vi "CRYGraph Intensity Window.vi"() -> ()   [LabVIEW 2013]
uses:
  <vilib>/Utility/miscctls.llb/LVPoint32TypeDef.ctl
  Control/CRYIntensity Property.ctl
  Control/CRYFlag Cluster.ctl
  <vilib>/Utility/miscctls.llb/LVRowAndColumnTypeDef.ctl
  <vilib>/Utility/miscctls.llb/LVPositionTypeDef.ctl
  SubVI/CRYData View Global.vi
  SubVI/CRYMain Sub Window Global.vi
  CRYCurveLibrary/Global/CRYCurve Library Global.vi
panel:
  out "Legend Ref":refnum<vi>
  in  "LoadFinish":bool
  in  "ScaleFitY":bool
  in  "ScaleFitX":bool
  in  "ToolbarUpdate":bool
  in  "OpenProperty":bool
  out "PropertyTab":string
  in  "RampShow":bool
  out "Intensity Property":T1 {"Type" items=["Rectangle"=0, "Hanning"=1, "Hamming"=2, "Blackman-Harris"=3, "Exact Blackman"=4, "Blackman"=5, "Flat Top"=6, "4 Term B-Harris"=7, "7 Term B-Harris"=8, "Low Sidelobe"=9, "Blackman Nuttall"=11, "Triangle"=30, "Bartlett-Hanning"=31, "Bohman"=32, "Parzen"=33, "Welch"=34, "Kaiser"=60, "Dolph-Chebyshev"=61, "Gaussian"=62]}
  in  "PaletteShow":bool
  in  "FitPanes":bool
  out "Graph Ref":refnum<vi>
  out "Repaint Watermark":i32
  out "Event Name":string
  out "ReportDrop":bool
  out "DirectionKey":bool
  out "PreviewGraph Ref":refnum<vi>
  in  "AxisChange":bool
  in  "RemoveOne":bool
  out "ScaleMin":dbl
  out "ScaleMax":dbl
  out "ScrollTick Ref":refnum<vi>
  out "Scrollbar Ref":refnum<vi>
  in  "PreviewShow":bool
  in  "CursorColor":bool
  out "NewCursIdx":u32
  out "Test":string
  in  "OldCursIdx":u32
  out "Queue Name":string
  in  "StateOut":bool
  in  "Cursor Waves":string[](array[string])
  out "Cursor Coords":T2
  in  "CursorPlot":bool
  out "Cursor Ref":refnum<vi>
  in  "CursorShow":bool
  out "IntensityGraph":dbl[][](graph)
  out "Title Name":string
  out "OldRow":i32
  out "TotalPlot":u32
  out "Graph Number":i32
  in  "stop":bool
  out "PreviewGraph":cluster{"xo":dbl, "dx":dbl, dbl[]}[](graph)
  in  "CursorEnabled":bool
  in  "Scrollbar":dbl(c297)
  in  "ScrollTick":dbl(slide) scale=0.0..1.0 scale format="%-#3.2p"
  in  "Cursor":string[][](table)
  in  "LegendShow":bool
  in  "Ramp":u16(ring)
  in  "Legend":i32(listbox)
  in  "GraphType":string
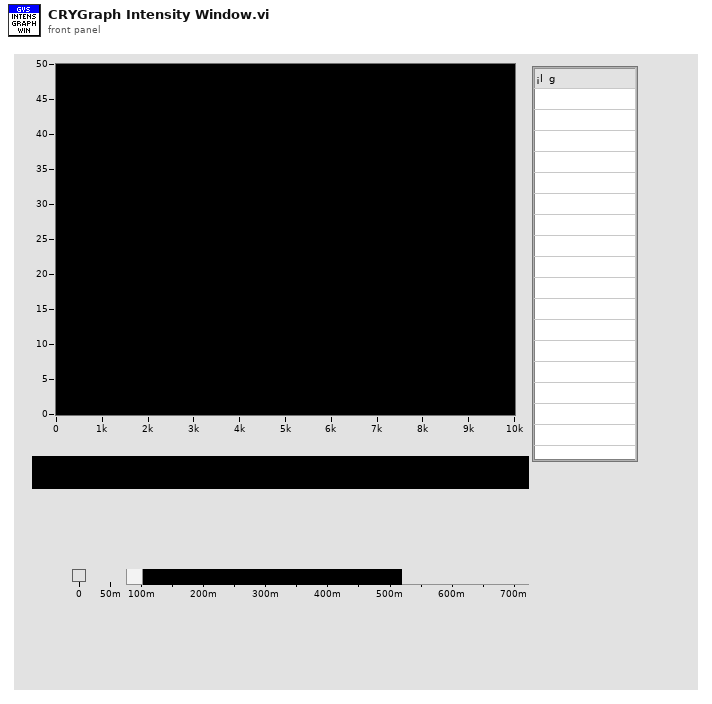
[diagram p1: front panel]
types:
  T1 = typedef "CRYIntensity Property.ctl" = cluster{"Time Steps":i32, "Frequency Bins":i32, "Type":u32, "Length":i32, "Map Type":enum16{"fire", "rainbow", "grey", "inverse grey", "ice", "original"}}
  T2 = typedef "LVPoint32TypeDef.ctl" = cluster{"Horizontal":i32, "Vertical":i32}
  T3 = typedef "CRYFlag Cluster.ctl" = cluster{"LegendShow":bool, "CellClick":bool, "Total Number":bool, "ScaleFitX":bool, "ScaleFitY":bool, "MapModeX":u8, "MapModeY":u8, "CursorShow":bool, "MagnitudeShow":bool, "PreviewShow":bool, "CursorEnabled":bool, "IntensityShow":bool, "PaletteShow":bool, "PhaseShow":bool, "XYShow":bool, "FrequencyShow":bool, "LegendVScrollShow":bool, "FrequencyVScrollShow":bool}
  T4 = typedef "LVPositionTypeDef.ctl" = cluster{"Left":i32, "Top":i32}
  T5 = typedef "LVRowAndColumnTypeDef.ctl" = cluster{"Row":i32, "Column":i32}
  T6 = typedef "CRYGraph Event.ctl" = cluster{"EvenName":string, "TitleName":string, "GraphName":string, "GraphType":string, "Data":variant, "Queue Name":string, "DataView Number":i32}
  T7 = enum16{"fire", "rainbow", "grey", "inverse grey", "ice", "original"}
  T8 = enum16{"No Scaling", "Scale All Objects", "Scale Single Object"}
  T9 = typedef "LVRectTypeDef.ctl" = cluster{"Left":i16, "Top":i16, "Right":i16, "Bottom":i16}
  T10 = typedef "LVBoundsTypeDef.ctl" = cluster{"Width":u32, "Height":u32}
  T11 = typedef "CRYWaveform Cluster.ctl" = cluster{"Waveform":cluster{"X0":dbl, "dX":dbl, "Y":sgl[]}, "X data":u16, "Y data":u16, "Y axis":u16, "X unit":string, "Y unit":string, "Y dB ref":dbl, "display Y":bool, "display X":bool, "Overload?":bool, "Test Info":string, "Step No.":i32, "Name":string, "protected":bool, "Sqc history":string[], "Signal Channel ID":i32, "Plot Settings":cluster{"Color":u32, "Interpolation":u8, "Point Style":u8, "Line Style":u8, "Point Color":u32, "Line Width":u8, "Bar Plot Style":u8, "Fill To":i16}, "AutoProtect":bool}
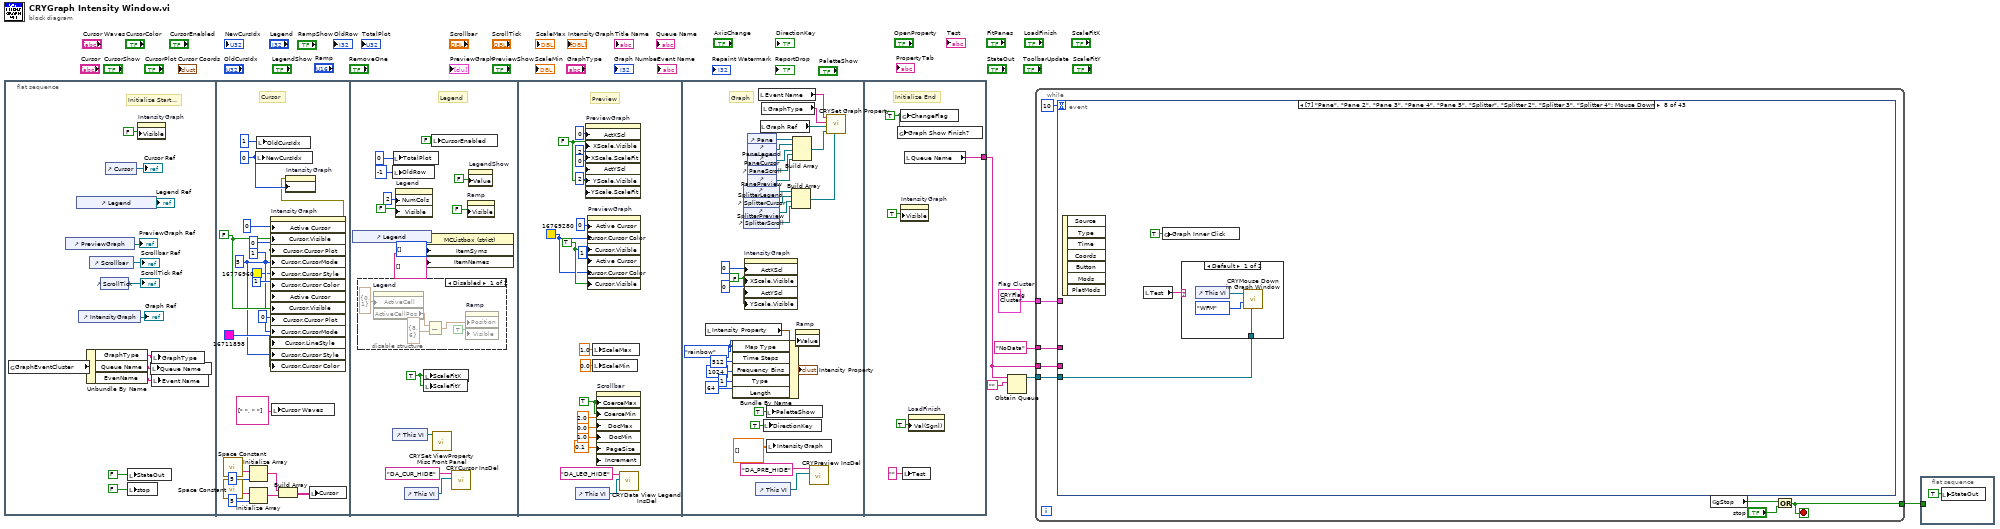
[diagram p0: block diagram]
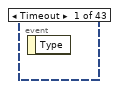
[diagram p3: hidden frame]
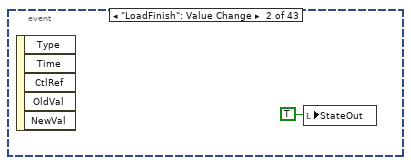
[diagram p4: hidden frame]
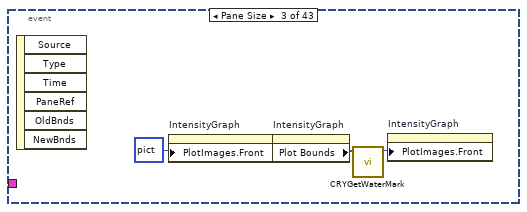
[diagram p5: hidden frame]
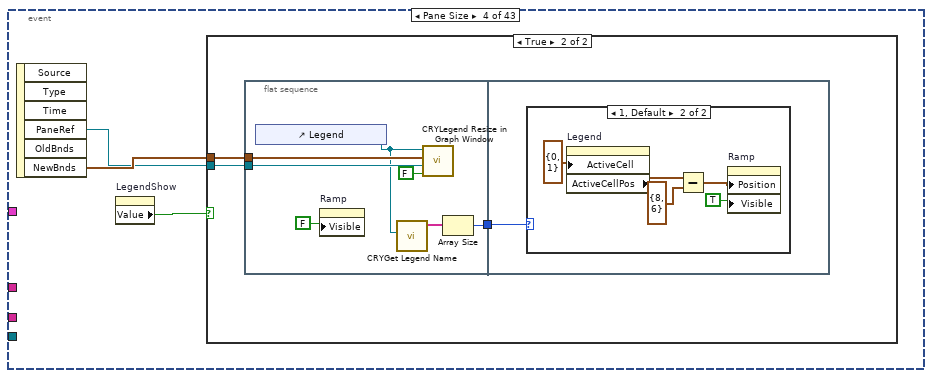
[diagram p6: hidden frame]
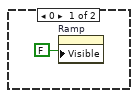
[diagram p8: hidden frame]
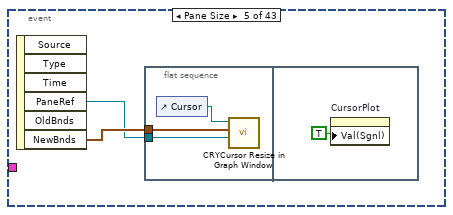
[diagram p9: hidden frame]
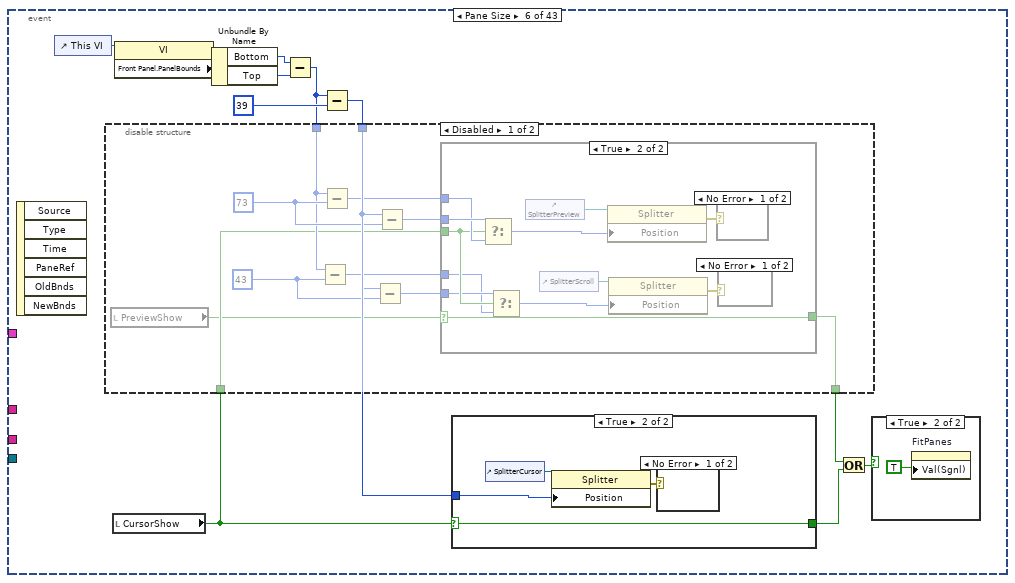
[diagram p10: hidden frame]
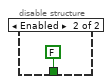
[diagram p14: hidden frame]
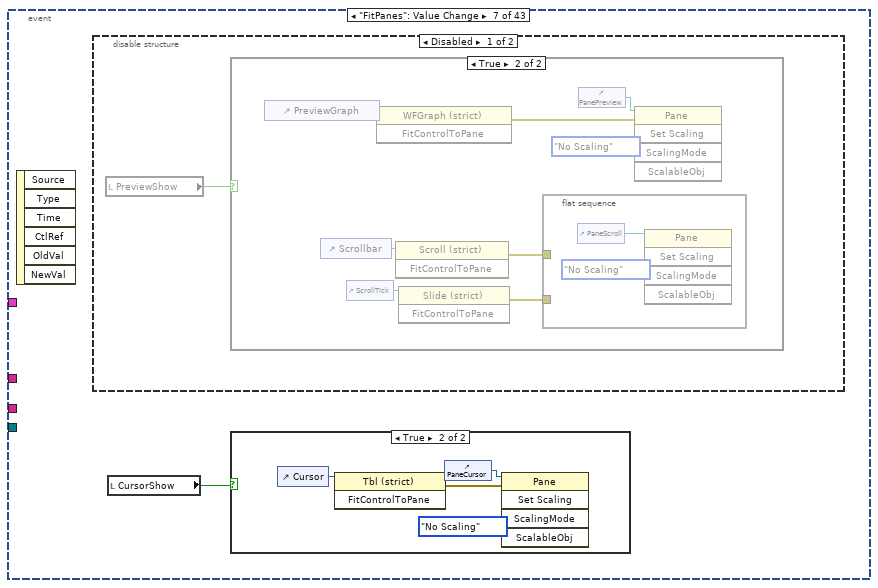
[diagram p18: hidden frame]
diagram:
  w4 = T3 {"LegendShow"=FALSE, "CellClick"=FALSE, "Total Number"=FALSE, "ScaleFitX"=FALSE, "ScaleFitY"=FALSE, "MapModeX"=0, "MapModeY"=0, "CursorShow"=FALSE, "MagnitudeShow"=FALSE, "PreviewShow"=FALSE, "CursorEnabled"=FALSE, "IntensityShow"=FALSE, "PaletteShow"=FALSE, "PhaseShow"=FALSE, "XYShow"=FALSE, "FrequencyShow"=FALSE, "LegendVScrollShow"=FALSE, "FrequencyVScrollShow"=FALSE}  # Flag Cluster
  n1 = flat-sequence {
    tunnel: [w107] -> w2
    frame #0 {
      # "Initialize Start..."
      n2 = global read "CRYData View Global.vi" "GraphEventCluster"() -> (w8:T6)
      n3 = control-ref of="PreviewGraph"() -> (→"PreviewGraph Ref":refnum<vi>)
      n4 = control-ref of="Legend"() -> (→"Legend Ref":refnum<vi>)
      n5 = control-ref of="IntensityGraph"() -> (→"Graph Ref":refnum<vi>)
      n6 = Unbundle By Name(w8) -> ("GraphType"=w10:string, "Queue Name"=w9:string, "EvenName"=w11:string)
      n7 = control-ref of="Scrollbar"() -> (→"Scrollbar Ref":refnum<vi>)
      n8 = control-ref of="ScrollTick"() -> (→"ScrollTick Ref":refnum<vi>)
      n9 = control-ref of="Cursor"() -> (→"Cursor Ref":refnum<vi>)
      n10 = local write "StateOut"(FALSE ("StateOut")) -> ()
      n11 = local write "stop"(FALSE ("stop")) -> ()
      n12 = property on="IntensityGraph" class="IntGraph (strict)"("Visible"=FALSE) -> ()  [unwired: 2 in, 2 out]
      n13 = local write "Queue Name"(w9) -> ()
      n14 = local write "GraphType"(w10) -> ()
      n15 = local write "Event Name"(w11) -> ()
    }
    frame #1 {
      w23 = u32 0 ("Active Cursor")
      w20 = u8 5 ("Cursor.Cursor Style")
      w26 = u32 1 ("Cursor.Cursor Mode")
      w27 = 0 ("Cursor.Cursor Plot")
      w28 = FALSE ("Cursor.Visible")
      # "Cursor"
      n16 = call <vilib>:"Space Constant.vi"() -> ("String"=w32:string)
      n17 = call <vilib>:"Space Constant.vi"() -> ("String"=w37:string)
      n18 = Initialize Array(w32, 5 ("dimension size")) -> (w34:string[])
      n19 = Initialize Array(w37, 5 ("dimension size")) -> (w38:string[])
      n20 = local write "NewCursIdx"(w23) -> ()
      n21 = local write "OldCursIdx"(u32 1 ("OldCursIdx")) -> ()
      n22 = property on="IntensityGraph" class="IntGraph (strict)"("Active Cursor"=u32 0, "Cursor.Visible"=w28, "Cursor.Cursor Plot"=w27, "Cursor.CursorMode"=w26, "Cursor.Cursor Style"=w20, "Cursor.Cursor Color"=u32 16776960, "Active Cursor"=u32 1, "Cursor.Visible"=w28, "Cursor.Cursor Plot"=w27, "Cursor.CursorMode"=w26, "Cursor.LineStyle"=u8 0 ("Cursor.Line Style"), "Cursor.Cursor Style"=w20, "Cursor.Cursor Color"=u32 16711898) -> (error out=w22:errorcluster)  [unwired: 2 in, 1 out]
      n23 = local write "Cursor Waves"(string[] [" ", " "] ("Cursor Waves")) -> ()
      n24 = Build Array(w34, w38) -> (w35:string[][])
      n25 = property on="IntensityGraph" class="IntGraph (strict)"(error in=w22, "Active Cursor"=w23) -> ()  [unwired: 1 in, 2 out]
      n26 = local write "Cursor"(w35) -> ()
    }
    frame #2 {
      w40 = TRUE ("ScaleFitX")
      # "Legend"
      n27 = control-ref of="Legend"() -> (w53:refnum<vi>)
      n28 = disable-structure shown="Disabled" {
        frame Disabled {
          n29 = property on="Legend" class="MCListbox (strict)"("ActiveCell"=T5 {"Row"=0, "Column"=1} ("Active Cell:Active Cell")) -> ("ActiveCellPos"=w54:T4)  [unwired: 2 in, 2 out]
          n30 = Subtract(x=w54, y=T4 {"Left"=8, "Top"=6}) -> (x-y=w57:T4)
          n31 = property on="Ramp" class="Ring (strict)"("Position"=w57, "Visible"=TRUE) -> ()  [unwired: 2 in, 2 out]
        }
        frame Enabled {
        }
      }
      n32 = local write "OldRow"(-1 ("OldRow 2")) -> ()
      n33 = control-ref of="This VI"() -> (w42:refnum<vi>)
      n34 = local write "TotalPlot"(u32 0 ("TotalPlot")) -> ()
      n35 = property on="Legend" class="MCListbox (strict)"("NumCols"=u32 2 ("Number of Columns"), "Visible"=FALSE) -> ()  [unwired: 2 in, 2 out]
      n36 = control-ref of="This VI"() -> (w44:refnum<vi>)
      n37 = local write "ScaleFitX"(w40) -> ()
      n38 = local write "ScaleFitY"(w40) -> ()
      n39 = property on="Property Node" class="MCListbox (strict)"(reference=w53, "ItemSyms"=i32[] [] ("Item Symbols"), "ItemNames"=string[][] [] ("Item Names")) -> ()  [unwired: 1 in, 2 out]
      n40 = local write "CursorEnabled"(FALSE ("CursorEnabled")) -> ()
      n41 = call "CRYSet ViewProperty Misc Front Panel.vi"("Vi Ref"=w42) -> ()  [unwired: 11 in]
      n42 = call "CRYCursor InsDel.vi"("Graph VI Ref"=w44, "sAction"="DA_CUR_HIDE" ("Action Type")) -> ()  [unwired: 10 in]
      n43 = property on="Ramp" class="Ring (strict)"("Visible"=FALSE) -> ()  [unwired: 2 in, 2 out]
      n44 = property on="LegendShow" class="Bool (strict)"("Value"=FALSE ("Visible")) -> ()  [unwired: 2 in, 2 out]
    }
    frame #3 {
      w64 = u32 16769280
      w65 = TRUE ("Cursor.Visible")
      w60 = FALSE ("X Scale.Visible")
      w76 = TRUE ("Coerce Maximum Value")
      # "Preview"
      n45 = control-ref of="This VI"() -> (w62:refnum<vi>)
      n46 = property on="PreviewGraph" class="WFGraph (strict)"("ActXScl"=0 ("Active X Scale"), "XScale.Visible"=w60, "XScale.ScaleFit"=u8 2 ("X Scale.Scale Fit"), "ActYScl"=0 ("Active Y Scale"), "YScale.Visible"=w60, "YScale.ScaleFit"=u8 2 ("Y Scale.Scale Fit")) -> ()  [unwired: 2 in, 2 out]
      n47 = property on="PreviewGraph" class="WFGraph (strict)"("Active Cursor"=u32 0, "Cursor.Cursor Color"=w64, "Cursor.Visible"=w65, "Active Cursor"=u32 1, "Cursor.Cursor Color"=w64, "Cursor.Visible"=w65) -> ()  [unwired: 2 in, 2 out]
      n48 = local write "ScaleMax"(1.0 ("ScaleMax")) -> ()
      n49 = local write "ScaleMin"(0.0 ("ScaleMin")) -> ()
      n50 = property on="Scrollbar" class="Scroll (strict)"("CoerceMax"=w76, "CoerceMin"=w76, "DocMax"=2.0 ("Doc Max"), "DocMin"=0.0 ("Doc Min"), "PageSize"=1.0 ("Page Size"), "Increment"=0.1) -> ()  [unwired: 2 in, 2 out]
      n51 = call "CRYData View Legend InsDel.vi"("Graph VI Ref"=w62, "sAction"="DA_LEG_HIDE" ("Action Type")) -> ()  [unwired: 2 in, 8 out]
    }
    frame #4 {
      w77 = FALSE ("X Scale.Visible")
      w81 = T7."rainbow" ("Map Type")
      # "Graph"
      n52 = local read "Intensity Property"() -> (w87:T1)
      n53 = Bundle By Name(cluster=w87, "Map Type"=w81, "Time Steps"=512, "Frequency Bins"=1024, "Type"=u32 1, "Length"=64) -> (→"Intensity Property":T1)
      n54 = control-ref of="SplitterLegend"() -> (w103:refnum<vi>)
      n55 = control-ref of="SplitterCursor"() -> (w102:refnum<vi>)
      n56 = control-ref of="SplitterPreview"() -> (w101:refnum<vi>)
      n57 = control-ref of="SplitterScroll"() -> (w100:refnum<vi>)
      n58 = property on="IntensityGraph" class="IntGraph (strict)"("ActXScl"=0 ("Active X Scale"), "XScale.Visible"=w77, "ActYScl"=0 ("Active Y Scale"), "YScale.Visible"=w77) -> ()  [unwired: 2 in, 2 out]
      n59 = control-ref of="Pane"() -> (w99:refnum<vi>)
      n60 = control-ref of="PaneLegend"() -> (w95:refnum<vi>)
      n61 = control-ref of="PaneCursor"() -> (w98:refnum<vi>)
      n62 = control-ref of="PaneScroll"() -> (w97:refnum<vi>)
      n63 = control-ref of="PanePreview"() -> (w96:refnum<vi>)
      n64 = control-ref of="This VI"() -> (w104:refnum<vi>)
      n65 = local read "Event Name"() -> (w89:string)
      n66 = local read "Graph Ref"() -> (w91:refnum<vi>)
      n67 = local read "GraphType"() -> (w90:string)
      n68 = local write "DirectionKey"(TRUE ("ScanCode")) -> ()
      n69 = local write "PaletteShow"(TRUE ("PaletteShow")) -> ()
      n70 = local write "IntensityGraph"(dbl[][] [] ("Graph")) -> ()
      n71 = Build Array(w103, w102, w101, w100) -> (w93:refnum<vi>[])
      n72 = Build Array(w99, w95, w98, w97, w96) -> (w94:refnum<vi>[])
      n73 = property on="Ramp" class="Ring (strict)"("Value"=w81) -> ()  [unwired: 2 in, 2 out]
      n74 = call "CRYPreview InsDel.vi"("Graph VI Ref"=w104, "sAction"="DA_PRE_HIDE" ("Action Type")) -> ()  [unwired: 10 in]
      n75 = call "CRYSet Graph Property.vi"("Splitters"=w93, "Panes"=w94, "Graph Ref"=w91, "Graph Type"=w90, "Event Name"=w89) -> ()  [unwired: 7 in]
    }
    frame #5 {
      w110 = TRUE ("ChangeFlag")
      # "Initialize End"
      n76 = global write "CRYData View Global.vi" "Graph Show Finish?"(w110) -> ()
      n77 = global write "CRYData View Global.vi" "ChangeFlag"(w110) -> ()
      n78 = property on="IntensityGraph" class="IntGraph (strict)"("Visible"=TRUE) -> ()  [unwired: 2 in, 2 out]
      n79 = local write "Test"("" ("Test")) -> ()
      n80 = local read "Queue Name"() -> (w107:string)
      n81 = property on="LoadFinish" class="Bool (strict)"("Val(Sgnl)"=TRUE ("Value (Signaling)")) -> ()  [unwired: 2 in, 2 out]
    }
  }
  n82 = Obtain Queue(name (unnamed)=w2, element data type="") -> (queue out=w6:refnum<queue>)  [unwired: 3 in, 2 out]
  n83 = while {
    tunnel: w6 -> [w118]
    tunnel: w4 -> [w116]
    tunnel: "NoData" ("input 2") -> [w113]
    tunnel: w2 -> [w112]
    tunnel: [w111] -> w1
    stop <- w111 stop-if-true
    n84 = event shown="[7] \"Pane\", \"Pane 2\", \"Pane 3\", \"Pane 4\", \"Pane 5\", \"Splitter\", \"Splitter 2\", \"Splitter 3\", \"Splitter 4\": Mouse Down" {
      selector: _ -> [_ _ _ _ _ _ _ _ _ _ _ _ _ _ _ _ _ _ _ _ _ _ _ _ _ _ _ _ _ _ _ _ _ _ _ _ _ _ _ _ _ _ _]
      dyn-events: _ -> [_ _ _ _ _ _ _ _ _ _ _ _ _ _ _ _ _ _ _ _ _ _ _ _ _ _ _ _ _ _ _ _ _ _ _ _ _ _ _ _ _ _ _]
      timeout: 10 -> [_ _ _ _ _ _ _ _ _ _ _ _ _ _ _ _ _ _ _ _ _ _ _ _ _ _ _ _ _ _ _ _ _ _ _ _ _ _ _ _ _ _ _]
      tunnel: w118 -> [_ _ _ _ _ _ _ w210 _ w243 _ w373 _ w410 _ _ _ _ _ _ _ _ _ _ w556 _ _ _ _ _ _ w643 _ _ w656 _ _ _ _ _ _ _ _]
      tunnel: w116 -> [_ _ _ _ _ _ _ _ w227 _ w355 _ w395 _ _ _ _ _ _ _ _ _ _ _ _ _ _ _ _ _ _ _ _ _ _ _ _ _ _ _ _ _ _]
      tunnel: w113 -> [_ _ _ _ _ _ _ _ _ w245 _ _ _ w409 _ _ _ _ _ _ _ _ _ _ _ _ _ _ _ _ _ _ _ _ _ _ _ _ _ _ _ _ _]
      tunnel: w112 -> [_ _ _ _ _ _ _ _ w220 w244 _ _ _ _ _ _ _ _ _ _ _ _ _ _ _ _ _ _ _ _ _ _ _ _ _ _ _ _ _ _ _ _ _]
      event Timeout {
        n85 = event-data() -> ()  [unwired: 2 out]
      }
      event "LoadFinish": Value Change {
        n86 = event-data() -> ()  [unwired: 6 out]
        n87 = local write "StateOut"(TRUE ("StateOut")) -> ()
      }
      event Pane Size {
        n88 = event-data() -> ()  [unwired: 7 out]
        n89 = property on="IntensityGraph" class="IntGraph (strict)"("PlotImages.Front"=picture data[5B] ("Plot Images:Front")) -> (error out=w120:errorcluster)  [unwired: 2 in, 1 out]
        n90 = property on="IntensityGraph" class="IntGraph (strict)"(error in=w120) -> ("Plot Bounds"=w122:T9)  [unwired: 1 in, 2 out]
        n91 = call "CRYGetWaterMark.vi"("Plot Area Bounds"=w122) -> ("WaterMark Image"=w121:picture)  [unwired: 3 in, 7 out]
        n92 = property on="IntensityGraph" class="IntGraph (strict)"("PlotImages.Front"=w121) -> ()  [unwired: 2 in, 2 out]
      }
      event Pane Size {
        n93 = event-data() -> ("PaneRef"=w125:refnum<vi>, "NewBnds"=w126:T9)  [unwired: 5 out]
        n94 = property on="LegendShow" class="Bool (strict)"() -> ("Value"=w124:bool)  [unwired: 2 in, 2 out]
        n95 = case shown="True" w124 {
          tunnel: w126 -> [_ w128]
          tunnel: w125 -> [_ w127]
          frame False {
          }
          frame True {
            n96 = flat-sequence {
              tunnel: w128 -> [w136]
              tunnel: w127 -> [w135]
              tunnel: [w131] -> w129
              tunnel: w129 -> [w137]
              frame #0 {
                n97 = control-ref of="Legend"() -> (w132:refnum<vi>)
                n98 = property on="Ramp" class="Ring (strict)"("Visible"=FALSE) -> ()  [unwired: 2 in, 2 out]
                n99 = call "CRYGet Legend Name.vi"("MCListbox Refnum"=w132) -> ("Names Out"=w133:string[])  [unwired: 10 in]
                n100 = call "CRYLegend Resize in Graph Window.vi"("VScrollShow"=FALSE, "Pane Ref"=w135, "input cluster"=w136, "Legend"=w132) -> ()  [unwired: 8 out]
                n101 = Array Size(array=w133) -> (size(s)=w131:i32)
              }
              frame #1 {
                n102 = case shown="1, Default" w137 {
                  frame 0 {
                    n103 = property on="Ramp" class="Ring (strict)"("Visible"=FALSE) -> ()  [unwired: 2 in, 2 out]
                  }
                  frame 1, Default {
                    n104 = property on="Legend" class="MCListbox (strict)"("ActiveCell"=T5 {"Row"=0, "Column"=1} ("Active Cell:Active Cell")) -> ("ActiveCellPos"=w143:T4)  [unwired: 2 in, 2 out]
                    n105 = Subtract(x=w143, y=T4 {"Left"=8, "Top"=6}) -> (x-y=w141:T4)
                    n106 = property on="Ramp" class="Ring (strict)"("Position"=w141, "Visible"=TRUE) -> ()  [unwired: 2 in, 2 out]
                  }
                }
              }
            }
          }
        }
      }
      event Pane Size {
        n107 = event-data() -> ("PaneRef"=w144:refnum<vi>, "NewBnds"=w145:T9)  [unwired: 5 out]
        n108 = flat-sequence {
          tunnel: w145 -> [w148]
          tunnel: w144 -> [w146]
          frame #0 {
            n109 = control-ref of="Cursor"() -> (w147:refnum<vi>)
            n110 = call "CRYCursor Resize in Graph Window.vi"("Pane Ref"=w146, "input cluster"=w148, "Graph Cursor Ref"=w147) -> ()  [unwired: 9 in]
          }
          frame #1 {
            n111 = property on="CursorPlot" class="Bool (strict)"("Val(Sgnl)"=TRUE ("Value (Signaling)")) -> ()  [unwired: 2 in, 2 out]
          }
        }
      }
      event Pane Size {
        n112 = event-data() -> ()  [unwired: 7 out]
        n113 = control-ref of="This VI"() -> (w153:refnum<vi>)
        n114 = local read "CursorShow"() -> (w150:bool)
        n115 = property class="VI"(reference=w153) -> ("Front Panel.PanelBounds"=w154:T9)  [unwired: 1 in, 2 out]
        n116 = Unbundle By Name(w154) -> ("Bottom"=w151:i16, "Top"=w152:i16)
        n117 = Subtract(x=w151, y=w152) -> (x-y=w155:i16)
        n118 = Subtract(x=w155, y=39) -> (x-y=w160:i32)
        n119 = disable-structure shown="Disabled" {
          disable-tunnel: w160 -> [w168 _]
          disable-tunnel: [w166 FALSE] -> w156
          disable-tunnel: w155 -> [w163 _]
          disable-tunnel: w150 -> [w162 _]
          frame Disabled {
            w169 = 43
            w167 = 73
            n120 = local read "PreviewShow"() -> (w161:bool)
            n121 = Subtract(x=w163, y=w169) -> (x-y=w165:i32)
            n122 = Subtract(x=w163, y=w167) -> (x-y=w164:i32)
            n123 = Subtract(x=w168, y=w169) -> (x-y=w171:i32)
            n124 = Subtract(x=w168, y=w167) -> (x-y=w170:i32)
            n125 = case shown="True" w161 {
              selector: w161 -> [w172 w182]
              tunnel: w164 -> [_ w180]
              tunnel: w165 -> [_ w176]
              tunnel: [w172 w182] -> w166
              tunnel: w162 -> [_ w178]
              tunnel: w170 -> [_ w181]
              tunnel: w171 -> [_ w177]
              frame False {
              }
              frame True {
                n126 = Select(t=w181, s=w178, f=w180) -> (s? t:f=w179:i32)
                n127 = Select(t=w177, s=w178, f=w176) -> (s? t:f=w175:i32)
                n128 = control-ref of="SplitterPreview"() -> (w174:refnum<vi>)
                n129 = control-ref of="SplitterScroll"() -> (w173:refnum<vi>)
                n130 = property class="Splitter"(reference=w174, "Position"=w179) -> (error out=w184:errorcluster)  [unwired: 1 in, 1 out]
                n131 = property class="Splitter"(reference=w173, "Position"=w175) -> (error out=w183:errorcluster)  [unwired: 1 in, 1 out]
                n132 = case shown="No Error" w184 {
                  frame No Error {
                  }
                  frame Error {
                  }
                }
                n133 = case shown="No Error" w183 {
                  frame No Error {
                  }
                  frame Error {
                  }
                }
              }
            }
          }
          frame Enabled {
          }
        }
        n134 = case shown="True" w150 {
          selector: w150 -> [w187 w189]
          tunnel: w160 -> [_ w191]
          tunnel: [w187 w189] -> w157
          frame False {
          }
          frame True {
            n135 = control-ref of="SplitterCursor"() -> (w188:refnum<vi>)
            n136 = property class="Splitter"(reference=w188, "Position"=w191) -> (error out=w190:errorcluster)  [unwired: 1 in, 1 out]
            n137 = case shown="No Error" w190 {
              frame No Error {
              }
              frame Error {
              }
            }
          }
        }
        n138 = Or(x=w156, y=w157) -> (x .or. y?=w158:bool)
        n139 = case shown="True" w158 {
          frame False {
          }
          frame True {
            n140 = property on="FitPanes" class="Bool (strict)"("Val(Sgnl)"=TRUE ("Value (Signaling)")) -> ()  [unwired: 2 in, 2 out]
          }
        }
      }
      event "FitPanes": Value Change {
        n141 = event-data() -> ()  [unwired: 7 out]
        n142 = disable-structure shown="Disabled" {
          frame Disabled {
            n143 = local read "PreviewShow"() -> (w193:bool)
            n144 = case shown="True" w193 {
              frame False {
              }
              frame True {
                n145 = control-ref of="PreviewGraph"() -> (w200:refnum<vi>)
                n146 = control-ref of="Scrollbar"() -> (w199:refnum<vi>)
                n147 = control-ref of="ScrollTick"() -> (w198:refnum<vi>)
                n148 = invoke class="WFGraph (strict)" method="FitControlToPane"(reference=w200) -> (error out=w197:errorcluster)  [unwired: 2 in, 2 out]
                n149 = invoke class="Scroll (strict)" method="FitControlToPane"(reference=w199) -> (error out=w196:errorcluster)  [unwired: 2 in, 2 out]
                n150 = invoke class="Slide (strict)" method="FitControlToPane"(reference=w198) -> (error out=w195:errorcluster)  [unwired: 2 in, 2 out]
                n151 = flat-sequence {
                  tunnel: w196 -> [_]
                  tunnel: w195 -> [_]
                  frame #0 {
                    n152 = control-ref of="PaneScroll"() -> (w202:refnum<vi>)
                    n153 = invoke class="Pane" method="Set Scaling"(reference=w202, "ScalingMode"=T8."No Scaling" ("Scaling Mode")) -> ()  [unwired: 3 in, 5 out]
                  }
                }
                n154 = control-ref of="PanePreview"() -> (w194:refnum<vi>)
                n155 = invoke class="Pane" method="Set Scaling"(reference=w194, error in=w197, "ScalingMode"=T8."No Scaling" ("Scaling Mode")) -> ()  [unwired: 2 in, 5 out]
              }
            }
          }
          frame Enabled {
          }
        }
        n156 = local read "CursorShow"() -> (w192:bool)
        n157 = case shown="True" w192 {
          frame False {
          }
          frame True {
            n158 = control-ref of="Cursor"() -> (w207:refnum<vi>)
            n159 = invoke class="Tbl (strict)" method="FitControlToPane"(reference=w207) -> (error out=w206:errorcluster)  [unwired: 2 in, 2 out]
            n160 = control-ref of="PaneCursor"() -> (w204:refnum<vi>)
            n161 = invoke class="Pane" method="Set Scaling"(reference=w204, error in=w206, "ScalingMode"=T8."No Scaling" ("Scaling Mode")) -> ()  [unwired: 2 in, 5 out]
          }
        }
      }
      event Mouse Down {
        n162 = event-data() -> ()  [unwired: 8 out]
        n163 = local read "Test"() -> (w209:string)
        n164 = global write "CRYCurve Library Global.vi" "Graph Inner Click"(TRUE ("Graph Inner Click")) -> ()
        n165 = case shown="Default" w209 {
          tunnel: w210 -> [w213 _]
          frame Default {
            n166 = control-ref of="This VI"() -> (w211:refnum<vi>)
            n167 = call "CRYMouse Down in Graph Window.vi"("Queue"=w213, "Selected Type"=enum16{"Curves", "Values", "Results", "WFM"}."WFM" ("Type"), "pGraph VI In"=w211) -> ()  [unwired: 3 in, 6 out]
          }
          frame "Test" {
          }
        }
      }
      event Shortcut Menu Activation? {
        n168 = event-data() -> ("MenuRef"=w229:refnum<k9>)  [unwired: 7 out]
        n169 = property on="IntensityGraph" class="IntGraph (strict)"() -> ("XScale.Mapping Mode"=w225:u8, "YScale.Mapping Mode"=w224:u8)  [unwired: 2 in, 2 out]
        n170 = local read "CursorEnabled"() -> (w222:bool)
        n171 = local read "LegendShow"() -> (w228:bool)
        n172 = local read "PreviewShow"() -> (w221:bool)
        n173 = local read "CursorShow"() -> (w223:bool)
        n174 = local read "PaletteShow"() -> (w216:bool)
        n175 = local read "ScaleFitX"() -> (w215:bool)
        n176 = local read "ScaleFitY"() -> (w214:bool)
        n177 = Bundle By Name(cluster=w227, "LegendShow"=w228, "ScaleFitX"=w215, "ScaleFitY"=w214, "MapModeX"=w225, "MapModeY"=w224, "CursorShow"=w223, "PreviewShow"=w221, "CursorEnabled"=w222, "PaletteShow"=w216) -> (w226:T3)
        n178 = local read "Test"() -> (w217:string)
        n179 = case shown="Default" w217 {
          tunnel: w220 -> [_ w235]
          tunnel: ["" ("sData Out") w234] -> w219
          tunnel: [TRUE ("bResult Out") w233] -> w218
          frame "Test" {
          }
          frame Default {
            n180 = local read "Graph Number"() -> (w232:i32)
            n181 = call "CRYGraph View Socket Client.vi"("sOption"="MENUOPTION", "nData"=w232, "sData"=w235, "sAction"="GET_GRAPHDATA") -> ("bResult Out"=w233:bool, "sData Out"=w234:string)  [unwired: 4 in, 2 out]
          }
        }
        n182 = case shown="True" w218 {
          tunnel: w229 -> [_ w242]
          tunnel: w226 -> [_ w240]
          tunnel: w219 -> [_ w239]
          frame False {
          }
          frame True {
            n183 = control-ref of="This VI"() -> (w238:refnum<vi>)
            n184 = call "CRYGraph Window Menu.vi"("MenuOption"=w239, "pGraph VI"=w238, "Flag Cluster"=w240, "Type"="INTENSITY", "Runtime Menu Ref In"=w242) -> ()  [unwired: 7 out]
          }
        }
        n185 = event-data() -> ()  [unwired: 1 in, 2 out]
      }
      event Shortcut Menu Selection (User) {
        n186 = event-data() -> ("ItemTag"=w246:string)  [unwired: 8 out]
        n187 = case shown="\"DA_SCALE_X_A\", \"DA_SCALE_X_L\", \"DA_SCALE_Y_A\", \"DA_SCALE_Y_L\"" w246 {
          selector: w246 -> [w248 _ w325 w351 _]
          tunnel: w245 -> [_ _ w319 _ _]
          tunnel: w244 -> [_ _ _ _ _]
          tunnel: w243 -> [_ _ w317 _ _]
          frame "DA_SCALE_X_A", "DA_SCALE_X_L", "DA_SCALE_Y_A", "DA_SCALE_Y_L" {
            n188 = case shown="\"DA_SCALE_X_A\", Default" w248 {
              selector: w248 -> [w252 w298 w299 w309]
              tunnel: [w252 w298 w299 w309] -> w247
              frame "DA_SCALE_X_A", Default {
                n189 = local read "ScaleFitX"() -> (w251:bool)
                n190 = Not(x=w251) -> (.not. x?=w250:bool)
                n191 = local write "ScaleFitX"(w250) -> ()
                n192 = Select(t=u8 2, s=w250, f=u8 0) -> (s? t:f=w253:u8)
                n193 = property on="IntensityGraph" class="IntGraph (strict)"("XScale.ScaleFit"=w253) -> (error out=w254:errorcluster)  [unwired: 2 in, 1 out]
                n194 = disable-structure shown="Disabled" {
                  disable-tunnel: w254 -> [w258 _]
                  disable-tunnel: w253 -> [w257 _]
                  frame Disabled {
                    n195 = property on="PreviewGraph" class="WFGraph (strict)"("XScale.ScaleFit"=w257) -> ()  [unwired: 2 in, 2 out]
                    n196 = case shown="2" w257 {
                      tunnel: w258 -> [_ _]
                      frame Default {
                      }
                      frame 2 {
                        n197 = property on="IntensityGraph" class="IntGraph (strict)"() -> ("XScale.Maximum"=w287:dbl, "XScale.Minimum"=w288:dbl)  [unwired: 2 in, 2 out]
                        n198 = property on="PreviewGraph" class="WFGraph (strict)"() -> ("XScale.Maximum"=w268:dbl, "XScale.Minimum"=w262:dbl)  [unwired: 2 in, 2 out]
                        n199 = Greater?(x=w262, y=w288) -> (0:w289:bool)
                        n200 = Less?(x=w268, y=w287) -> (x < y?=w286:bool)
                        n201 = Subtract(x=w268, y=w262) -> (x-y=w267:dbl)
                        n202 = Select(t=w268, s=w286, f=w287) -> (s? t:f=w263:dbl)
                        n203 = Select(t=w262, s=w289, f=w288) -> (s? t:f=w264:dbl)
                        n204 = Subtract(x=w264, y=w262) -> (x-y=w261:dbl)
                        n205 = Subtract(x=w263, y=w262) -> (x-y=w260:dbl)
                        n206 = property on="PreviewGraph" class="WFGraph (strict)"("Active Cursor"=u32 0, "Cursor.Cursor X"=w264, "Active Cursor"=u32 1, "Cursor.Cursor X"=w263) -> (error out=w285:errorcluster)  [unwired: 2 in, 1 out]
                        n207 = Divide(x=w261, y=w267) -> (x/y=w265:dbl)
                        n208 = Divide(x=w260, y=w267) -> (x/y=w266:dbl)
                        n209 = property on="Scrollbar" class="Scroll (strict)"() -> ("DocMax"=w274:dbl, "PageSize"=w280:dbl)  [unwired: 2 in, 2 out]
                        n210 = Subtract(x=w265, y=w266) -> (x-y=w272:dbl)
                        n211 = flat-sequence {
                          tunnel: w285 -> [_]
                          frame #0 {
                            n212 = control-ref of="This VI"() -> (w291:refnum<vi>)
                            n213 = call "CRYPlot Wave Graph Preview.vi"("sOption"="Move", "Graph VI Ref"=w291) -> ()  [unwired: 10 in]
                          }
                        }
                        n214 = Divide(x=w280, y=w272) -> (x/y=w271:dbl)
                        n215 = local read "ScaleMax"() -> (w270:dbl)
                        n216 = local read "ScaleMin"() -> (w269:dbl)
                        n217 = Add(x=w274, y=w271) -> (x+y=w273:dbl)
                        n218 = property on="Scrollbar" class="Scroll (strict)"("DocMin"=w273) -> ("DocMax"=w282:dbl, "DocMin"=w281:dbl)  [unwired: 2 in, 2 out]
                        n219 = Subtract(x=w270, y=w269) -> (x-y=w259:dbl)
                        n220 = Subtract(x=w265, y=w269) -> (x-y=w275:dbl)
                        n221 = Subtract(x=w282, y=w281) -> (x-y=w276:dbl)
                        n222 = Multiply(x=w275, y=w276) -> (x*y=w277:dbl)
                        n223 = Divide(x=w277, y=w259) -> (x/y=w278:dbl)
                        n224 = Add(x=w278, y=w281) -> (x+y=w279:dbl)
                        n225 = property on="Scrollbar" class="Scroll (strict)"("Value"=w279) -> ()  [unwired: 2 in, 2 out]
                      }
                    }
                  }
                  frame Enabled {
                  }
                }
              }
              frame "DA_SCALE_Y_A" {
                n226 = local read "ScaleFitY"() -> (w293:bool)
                n227 = Not(x=w293) -> (.not. x?=w292:bool)
                n228 = local write "ScaleFitY"(w292) -> ()
                n229 = Select(t=u8 2, s=w292, f=u8 0) -> (s? t:f=w295:u8)
                n230 = property on="IntensityGraph" class="IntGraph (strict)"("ActYScl"=0 ("Active Y Scale"), "YScale.ScaleFit"=w295) -> ()  [unwired: 2 in, 2 out]
              }
              frame "DA_SCALE_X_L" {
                n231 = property on="IntensityGraph" class="IntGraph (strict)"() -> ("XScale.Mapping Mode"=w300:u8)  [unwired: 2 in, 2 out]
                n232 = Equal?(x=w300, y=u8 0) -> (x = y?=w305:bool)
                n233 = Select(t=u8 1, s=w305, f=u8 0) -> (s? t:f=w301:u8)
                n234 = property on="IntensityGraph" class="IntGraph (strict)"("XScale.Mapping Mode"=w301) -> ()  [unwired: 2 in, 2 out]
              }
              frame "DA_SCALE_Y_L" {
                n235 = property on="IntensityGraph" class="IntGraph (strict)"("ActYScl"=0 ("Active Y Scale")) -> ("YScale.Mapping Mode"=w308:u8)  [unwired: 2 in, 2 out]
                n236 = Equal To 0?(x=w308) -> (x = 0?=w313:bool)
                n237 = Select(t=u8 1, s=w313, f=u8 0) -> (s? t:f=w310:u8)
                n238 = property on="IntensityGraph" class="IntGraph (strict)"("ActYScl"=0 ("Active Y Scale"), "YScale.Mapping Mode"=w310) -> ()  [unwired: 2 in, 2 out]
              }
            }
            n239 = case shown="\"DA_SCALE_X_A\", \"DA_SCALE_Y_A\"" w247 {
              frame Default {
              }
              frame "DA_SCALE_X_A", "DA_SCALE_Y_A" {
                n240 = property on="ToolbarUpdate" class="Bool (strict)"("Val(Sgnl)"=TRUE ("Value (Signaling)")) -> ()  [unwired: 2 in, 2 out]
              }
            }
          }
          frame "DA_EXPORT_EXCEL" {
            w315 = enum16{"Curves", "Values", "Results", "WFM"}."WFM" ("Type")
            n241 = control-ref of="Legend"() -> (w314:refnum<vi>)
            n242 = call "CRYGet Graph Data in Graph.vi"("Legend Refnum"=w314, "Type In"=w315) -> ("Rows"=w316:i32[])  [unwired: 2 in, 7 out]
            n243 = call "CRYExport to Excel.vi"("Rows"=w316, "Type"=w315) -> ()  [unwired: 2 in, 8 out]
          }
          frame Default {
            n244 = Search/Split String(string=w325, search string/char (-)="#") -> (substring before match=w320:string, match + rest of string=w323:string)  [unwired: 2 out]
            n245 = call "CRYPreUpdate Sequence.vi"("EventName"="CurLibUpdate") -> ()  [unwired: 15 in]
            n246 = Decimal String To Number(string=w323, offset=1) -> (number=w321:i32)  [unwired: 2 out]
            n247 = case shown="0, Default" w321 {
              selector: w321 -> [_ w338]
              tunnel: w320 -> [w328 w340]
              tunnel: w319 -> [_ _]
              tunnel: w317 -> [w332 w336]
              frame 0, Default {
                n248 = local read "GraphType"() -> (w326:string)
                n249 = local read "Graph Number"() -> (w333:i32)
                n250 = Equal?(x="DA_EXPORT_DOCUMENT" ("y"), y=w328) -> (x = y?=w331:bool)
                n251 = Select(t="ADD_DOC", s=w331, f=w328) -> (s? t:f=w327:string)
                n252 = Format Into String(w327, w326, w333, 0 ("input 3")) -> (resulting string=w334:string)  [unwired: 3 in, 1 out]
                n253 = Enqueue Element(queue=w332, element=w334) -> ()  [unwired: 1 in, 4 out]
              }
              frame 1..10 {
                n254 = flat-sequence {
                  tunnel: w340 -> [w343]
                  tunnel: [w343] -> w339
                  tunnel: w338 -> [w342]
                  tunnel: [w341] -> w337
                  tunnel: w339 -> [w347]
                  tunnel: w337 -> [w345]
                  tunnel: w336 -> [w344]
                  frame #0 {
                    n255 = call "CRYSet Graph Cluster Data.vi"("Graph Number"=w342) -> ("DataType"=w341:string)  [unwired: 2 in, 8 out]
                  }
                  frame #1 {
                    n256 = local read "Graph Number"() -> (w346:i32)
                    n257 = Format Into String(w347, w345, w346, 0 ("input 3")) -> (resulting string=w349:string)  [unwired: 3 in, 1 out]
                    n258 = Enqueue Element(queue=w344, element=w349) -> ()  [unwired: 1 in, 4 out]
                  }
                }
              }
            }
          }
          frame "DA_PAL_HIDE", "DA_PAL_VIEW" {
            n259 = Equal?(x=w351, y="DA_PAL_VIEW") -> (x = y?=w350:bool)
            n260 = property on="PaletteShow" class="Bool (strict)"("Val(Sgnl)"=w350) -> ()  [unwired: 2 in, 2 out]
          }
          frame "DA_REMOVE" {
            n261 = property on="RemoveOne" class="Bool (strict)"("Val(Sgnl)"=TRUE ("Value (Signaling)")) -> ()  [unwired: 2 in, 2 out]
          }
        }
      }
      event Shortcut Menu Activation? {
        n262 = event-data() -> ("MenuRef"=w356:refnum<k9>, "Coords"=w357:T2)  [unwired: 6 out]
        n263 = local read "LegendShow"() -> (w354:bool)
        n264 = case shown="True" w354 {
          selector: w354 -> [_ w359]
          tunnel: w357 -> [_ w370]
          tunnel: w356 -> [_ w368]
          tunnel: w355 -> [_ w364]
          frame False {
          }
          frame True {
            n265 = invoke on="Legend" class="MCListbox (strict)" method="Point To Row Column"("Point"=w370) -> ("CellPosition"=w371:T5)  [unwired: 6 in, 6 out]
            n266 = local read "TotalPlot"() -> (w362:u32)
            n267 = Unbundle By Name(w371) -> ("Row"=w358:i32)
            n268 = To Long Integer(number=w362) -> (32bit integer=w361:i32)
            n269 = Less?(x=w358, y=w361) -> (x < y?=w366:bool)
            n270 = local write "OldRow"(w358) -> ()
            n271 = Greater?(x=w362, y=u32 0) -> (0:w365:bool)
            n272 = property on="Legend" class="MCListbox (strict)"("Value"=w358) -> ()  [unwired: 2 in, 2 out]
            n273 = Bundle By Name(cluster=w364, "LegendShow"=w359, "CellClick"=w366, "Total Number"=w365) -> (w363:T3)
            n274 = control-ref of="This VI"() -> (w360:refnum<vi>)
            n275 = call "CRYGraph Window Menu.vi"("pGraph VI"=w360, "Flag Cluster"=w363, "Type"="LEGEND", "Runtime Menu Ref In"=w368) -> ()  [unwired: 1 in, 7 out]
          }
        }
        n276 = event-data() -> ()  [unwired: 1 in, 2 out]
      }
      event Shortcut Menu Selection (User) {
        n277 = event-data() -> ("ItemTag"=w374:string)  [unwired: 8 out]
        n278 = local read "Graph Number"() -> (w372:i32)
        n279 = case shown="\"DA_LEG_REMOVE\"" w374 {
          tunnel: w373 -> [_ w379 _ _]
          tunnel: w372 -> [_ w378 _ _]
          frame Default {
          }
          frame "DA_LEG_HIDE_1" {
            n280 = Format Into String("DA_LEG_HIDE" ("input 1"), "AAA" ("input 2"), w378, 0 ("input 3")) -> (resulting string=w380:string)  [unwired: 3 in, 1 out]
            n281 = Enqueue Element(queue=w379, element=w380) -> ()  [unwired: 1 in, 4 out]
          }
          frame "DA_LEG_REMOVE" {
            n282 = property on="RemoveOne" class="Bool (strict)"("Val(Sgnl)"=TRUE ("Value (Signaling)")) -> ()  [unwired: 2 in, 2 out]
          }
          frame "DA_LEG_INVERT" {
            n283 = local read "TotalPlot"() -> (w382:u32)
            n284 = for {
              N: w382 -> [_]
              tunnel: [w385] -> w383
              i -> [w386]
              w387 = 38
              w389 = 37
              n285 = property on="Legend" class="MCListbox (strict)"() -> ("ItemSyms"=w391:i32[])  [unwired: 2 in, 2 out]
              n286 = Index Array(array=w391, index=w386) -> (element=w390:i32)
              n287 = Equal?(x=w390, y=w389) -> ()  [unwired: 1 out]
              n288 = Equal?(x=w390, y=w387) -> (x = y?=w388:bool)
              n289 = Select(t=w389, s=w388, f=w387) -> (s? t:f=w392:i32)
              n290 = Replace Array Subset(array=w391, new element=w392, index=w386) -> (w393:i32[])
              n291 = property on="Legend" class="MCListbox (strict)"("ItemSyms"=w393) -> (error out=w385:errorcluster)  [unwired: 2 in, 1 out]
            }
            n292 = property on="AxisChange" class="Bool (strict)"(error in=w383, "Val(Sgnl)"=TRUE ("Value (Signaling)")) -> ()  [unwired: 1 in, 2 out]
          }
        }
      }
      event Shortcut Menu Activation? {
        n293 = event-data() -> ("MenuRef"=w396:refnum<k9>)  [unwired: 7 out]
        n294 = local read "CursorShow"() -> (w394:bool)
        n295 = case shown="True" w394 {
          selector: w394 -> [_ w397]
          tunnel: w396 -> [_ w400]
          tunnel: w395 -> [_ w399]
          frame False {
          }
          frame True {
            n296 = Bundle By Name(cluster=w399, "CursorShow"=w397) -> (w401:T3)
            n297 = control-ref of="This VI"() -> (w398:refnum<vi>)
            n298 = call "CRYGraph Window Menu.vi"("pGraph VI"=w398, "Flag Cluster"=w401, "Type"="CURSOR", "Runtime Menu Ref In"=w400) -> ()  [unwired: 1 in, 7 out]
          }
        }
        n299 = event-data() -> ()  [unwired: 2 in, 1 out]
      }
      event Shortcut Menu Selection (User) {
        n300 = event-data() -> ("ItemTag"=w405:string)  [unwired: 8 out]
        n301 = local read "Graph Number"() -> (w407:i32)
        n302 = Match Pattern(string=w405, regular expression="#" ("search string/char (-)")) -> (before substring=w404:string, after substring=w403:string)  [unwired: 1 in, 2 out]
        n303 = case shown="\"DA_CUR_HIDE_1\"" w404 {
          selector: w404 -> [_ w422 w438 _]
          tunnel: w410 -> [_ _ w436 w443]
          tunnel: w407 -> [_ _ w439 w445]
          tunnel: w409 -> [_ _ w437 w444]
          tunnel: w403 -> [w411 _ _ _]
          frame "DA_CUR_GOTO_CUR" {
            n304 = Decimal String To Number(string=w411) -> (number=w412:i32)  [unwired: 1 in, 2 out]
            n305 = case shown="0, 1" w412 {
              selector: w412 -> [_ w414]
              frame Default {
              }
              frame 0, 1 {
                n306 = flat-sequence {
                  tunnel: w414 -> [w416]
                  frame #0 {
                    n307 = Equal To 0?(x=w416) -> (x = 0?=w420:bool)
                    n308 = local write "NewCursIdx"(w416) -> ()
                    n309 = property on="IntensityGraph" class="IntGraph (strict)"("Active Cursor"=w416) -> ()  [unwired: 2 in, 2 out]
                    n310 = Select(t=1 ("OldCursIdx"), s=w420, f=0 ("OldCursIdx")) -> (s? t:f=w417:i32)
                    n311 = local write "OldCursIdx"(w417) -> ()
                  }
                  frame #1 {
                    n312 = property on="CursorColor" class="Bool (strict)"("Val(Sgnl)"=TRUE ("Value (Signaling)")) -> ()  [unwired: 2 in, 2 out]
                  }
                }
                n313 = control-ref of="IntensityGraph"() -> (w413:refnum<vi>)
                n314 = call "CRYGoto Cursor.vi"("Active Cursor"=w414, "Graph Ref"=w413, "Graph Type"="INTENSITY") -> ()  [unwired: 9 in]
              }
            }
          }
          frame "LINKTO" {
            n315 = Match Pattern(string=w422, regular expression="[0-1]_") -> (match substring=w426:string, after substring=w424:string)  [unwired: 1 in, 2 out]
            n316 = Decimal String To Number(string=w426) -> (number=w423:i32)  [unwired: 2 in, 1 out]
            n317 = case shown="0, 1" w423 {
              selector: w423 -> [w427 _]
              tunnel: w424 -> [w428 _]
              frame 0, 1 {
                n318 = control-ref of="Legend"() -> (w431:refnum<vi>)
                n319 = local read "Cursor Waves"() -> (w430:string[])
                n320 = control-ref of="IntensityGraph"() -> ()  [unwired: 1 out]
                n321 = call "CRYGet Legend Name.vi"("MCListbox Refnum"=w431) -> ("Names Out"=w432:string[])  [unwired: 10 in]
                n322 = Search 1D Array(1D array=w432, element=w428) -> (index of element=w433:i32)  [unwired: 1 in]
                n323 = Replace Array Subset(array=w430, new element=w428, index=w427) -> (w429:string[])
                n324 = case shown="0, Default" w433 {
                  selector: w433 -> [w434 _]
                  tunnel: w427 -> [w435 _]
                  frame 0, Default {
                    n325 = property on="IntensityGraph" class="IntGraph (strict)"("Active Cursor"=w435, "Cursor.Cursor Plot"=w434) -> ()  [unwired: 2 in, 2 out]
                  }
                  frame -1 {
                  }
                }
                n326 = local write "Cursor Waves"(w429) -> ()
              }
              frame Default {
              }
            }
          }
          frame Default {
            n327 = Format Into String(w438, w437, w439, 0 ("input 3")) -> (resulting string=w440:string)  [unwired: 3 in, 1 out]
            n328 = Enqueue Element(queue=w436, element=w440) -> ()  [unwired: 1 in, 4 out]
          }
          frame "DA_CUR_HIDE_1" {
            n329 = Format Into String("DA_CUR_HIDE" ("input 1"), w444, w445, 0 ("input 3")) -> (resulting string=w446:string)  [unwired: 3 in, 1 out]
            n330 = Enqueue Element(queue=w443, element=w446) -> ()  [unwired: 1 in, 4 out]
          }
        }
        n331 = call "CRYPreUpdate Sequence.vi"("EventName"="CurLibUpdate") -> ()  [unwired: 15 in]
      }
      event "PaletteShow": Value Change {
        n332 = event-data() -> ("NewVal"=w448:bool)  [unwired: 6 out]
        n333 = property on="IntensityGraph" class="IntGraph (strict)"("Palette Visible"=w448) -> ()  [unwired: 2 in, 2 out]
      }
      event "Cursor": Key Down; "Cursor": Key Repeat {
        n334 = event-data() -> ("ScanCode"=w449:i16)  [unwired: 10 out]
        n335 = disable-structure shown="Disabled" {
          disable-tunnel: [w454 0.1 ("XScale.MinorInc")] -> w451
          frame Disabled {
            n336 = local read "NewCursIdx"() -> (w458:u32)
            n337 = property on="IntensityGraph" class="IntGraph (strict)"("Active Cursor"=w458) -> ("Value"=w459:dbl[][], "Cursor.Cursor Plot"=w457:i32)  [unwired: 2 in, 2 out]
            n338 = property on="IntensityGraph" class="IntGraph (strict)"() -> ("XScale.MinorInc"=w455:dbl)  [unwired: 2 in, 2 out]
            n339 = Index Array(array=w459, index (row)=w457) -> (element=w453:dbl[])  [unwired: 1 in]
            n340 = Unbundle By Name(w453) -> ("dx"=w452)
            n341 = Greater Or Equal?(x=w455, y=w452) -> (x >= y?=w456:bool)
            n342 = Select(t=w455, s=w456, f=w452) -> (s? t:f=w454:dbl)
          }
          frame Enabled {
          }
        }
        n343 = case shown="75" w449 {
          tunnel: w451 -> [_ w466 w470]
          tunnel: [errorcluster {"status"=FALSE, "code"=0, "source"=""} ("error out") w464 w468] -> w450
          frame 0, Default {
            n344 = local write "DirectionKey"(FALSE ("ScanCode")) -> ()
          }
          frame 77 {
            n345 = property on="IntensityGraph" class="IntGraph (strict)"() -> ("Cursor.Cursor X"=w467:dbl)  [unwired: 2 in, 2 out]
            n346 = Add(x=w467, y=w466) -> (x+y=w465:dbl)
            n347 = property on="IntensityGraph" class="IntGraph (strict)"("Cursor.Cursor X"=w465) -> (error out=w464:errorcluster)  [unwired: 2 in, 1 out]
          }
          frame 75 {
            n348 = property on="IntensityGraph" class="IntGraph (strict)"() -> ("Cursor.Cursor X"=w471:dbl)  [unwired: 2 in, 2 out]
            n349 = Subtract(x=w471, y=w470) -> (x-y=w469:dbl)
            n350 = property on="IntensityGraph" class="IntGraph (strict)"("Cursor.Cursor X"=w469) -> (error out=w468:errorcluster)  [unwired: 2 in, 1 out]
          }
        }
        n351 = case shown="No Error" w450 {
          frame No Error {
            n352 = property on="CursorPlot" class="Bool (strict)"("Val(Sgnl)"=TRUE ("Value (Signaling)")) -> ()  [unwired: 2 in, 2 out]
          }
          frame Error {
          }
        }
      }
      event "Cursor": Mouse Down {
        n353 = event-data() -> ("CtlRef"=w475:refnum<vi>, "Coords"=w472:T2)  [unwired: 7 out]
        n354 = invoke class="Tbl (strict)" method="Point To Row Column"(reference=w475, "Point"=w472) -> ("CellPosition"=w474:T5)  [unwired: 4 in, 5 out]
        n355 = local write "Cursor Coords"(w472) -> ()
        n356 = Unbundle By Name(w474) -> ("Row"=w473:i32)
        n357 = flat-sequence {
          tunnel: w473 -> [w476]
          frame #0 {
            n358 = Equal To 0?(x=w476) -> (x = 0?=w480:bool)
            n359 = local write "NewCursIdx"(w476) -> ()
            n360 = property on="IntensityGraph" class="IntGraph (strict)"("Active Cursor"=w476) -> ()  [unwired: 2 in, 2 out]
            n361 = Select(t=1 ("OldCursIdx"), s=w480, f=0 ("OldCursIdx")) -> (s? t:f=w477:i32)
            n362 = local write "OldCursIdx"(w477) -> ()
          }
          frame #1 {
            n363 = property on="CursorColor" class="Bool (strict)"("Val(Sgnl)"=TRUE ("Value (Signaling)")) -> ()  [unwired: 2 in, 2 out]
          }
        }
      }
      event "Cursor": Value Change {
        n364 = event-data() -> ("OldVal"=w486:string[][], "NewVal"=w485:string[][])  [unwired: 5 out]
        n365 = local read "Cursor Coords"() -> (w483:T2)
        n366 = control-ref of="This VI"() -> (w484:refnum<vi>)
        n367 = call "CRYCursor move in Cursor Table.vi"("NewVal"=w485, "OldVal"=w486, "Cursor Coords"=w483, "pGraph VI"=w484) -> ("NewVal Out"=w482:string[][])  [unwired: 7 in]
        n368 = local write "Cursor"(w482) -> ()
      }
      event "CursorShow": Value Change {
        n369 = event-data() -> ("NewVal"=w487:bool)  [unwired: 6 out]
        n370 = flat-sequence {
          tunnel: w487 -> [w492]
          frame #0 {
            n371 = Select(t="DA_CUR_VIEW", s=w492, f="DA_CUR_HIDE") -> (s? t:f=w491:string)
            n372 = control-ref of="This VI"() -> (w488:refnum<vi>)
            n373 = call "CRYCursor InsDel.vi"("Graph VI Ref"=w488, "sAction"=w491) -> ()  [unwired: 10 in]
          }
          frame #1 {
            n374 = property on="ToolbarUpdate" class="Bool (strict)"("Val(Sgnl)"=TRUE ("Value (Signaling)")) -> ()  [unwired: 2 in, 2 out]
          }
        }
      }
      event "CursorPlot": Value Change {
        n375 = event-data() -> ()  [unwired: 7 out]
        n376 = local read "CursorShow"() -> (w494:bool)
        n377 = case shown="True" w494 {
          frame False {
          }
          frame True {
            n378 = control-ref of="IntensityGraph"() -> (w495:refnum<vi>)
            n379 = control-ref of="Cursor"() -> (w496:refnum<vi>)
            n380 = call "CRYPlot Cursor.vi"("Cursor Ref"=w496, "Graph Ref"=w495, "Graph Type"="INTENSITY") -> ()  [unwired: 9 in]
          }
        }
      }
      event "CursorColor": Value Change {
        n381 = event-data() -> ()  [unwired: 7 out]
        n382 = local read "NewCursIdx"() -> (w508:u32)
        n383 = local read "OldCursIdx"() -> (w509:u32)
        n384 = property on="IntensityGraph" class="IntGraph (strict)"("Active Cursor"=w509) -> ("Cursor.Cursor Color"=w501:u32)  [unwired: 2 in, 2 out]
        n385 = property on="IntensityGraph" class="IntGraph (strict)"("Active Cursor"=w508) -> ("Cursor.Cursor Color"=w500:u32)  [unwired: 2 in, 2 out]
        n386 = Bundle By Name(cluster=T5 {"Row"=0, "Column"=0} ("Active Cell:Active Cell"), "Row"=w508, "Column"=0) -> (w505:T5)
        n387 = Bundle By Name(cluster=T5 {"Row"=0, "Column"=0} ("Active Cell:Active Cell"), "Row"=w509, "Column"=0) -> (w502:T5)
        n388 = property on="Cursor" class="Tbl (strict)"("Active Cell"=w502, "CellFontColor"=w501, "Cell BG Color"=u32 16777226) -> ()  [unwired: 2 in, 2 out]
        n389 = property on="Cursor" class="Tbl (strict)"("Active Cell"=w505, "CellFontColor"=w500, "Cell BG Color"=u32 60927) -> ()  [unwired: 2 in, 2 out]
      }
      event "Legend": Mouse Down {
        n390 = event-data() -> ("CtlRef"=w512:refnum<vi>, "Coords"=w517:T2, "Button"=w516:u16)  [unwired: 6 out]
        n391 = local read "Test"() -> (w510:string)
        n392 = local read "TotalPlot"() -> (w513:u32)
        n393 = call "CRYData View Legend Plot OnOff.vi"("TotalPlot"=w513, "Button Info"=w516, "Mouse Point"=w517, "MCListbox Ref In"=w512) -> ("Active Row"=w511:i32, "Visible?"=w514:bool, "Click State"=w515:bool)  [unwired: 5 out]
        n394 = case shown="Default" w510 {
          tunnel: w512 -> [_ w522]
          tunnel: w511 -> [_ w520]
          frame "Test" {
          }
          frame Default {
            n395 = local read "GraphType"() -> (w521:string)
            n396 = Build Array(w520) -> (w519:i32[])
            n397 = call "CRYData View Legend Manipulate.vi"("sAction"="GetViewNumbyLegNum", "nData"=w519, "sData"=w521, "Legend Ref"=w522) -> ("nData Out"=w523:i32[])  [unwired: 6 in, 1 out]
            n398 = call "CRYGet Graph Name From Graph Type.vi"("Graph Type"=w521) -> ("Type"=w525:enum16{"Curves", "Values", "Results", "WFM"})  [unwired: 9 in, 1 out]
            n399 = call "CRYTree Global Manipulate.vi"("Type In"=w525) -> ("Tree/Curve Tree"=w524:refnum<vi>)  [unwired: 7 in, 3 out]
            n400 = call "CRYTree Manuplate.vi"("sAction"="SetActiveNumbers", "nData"=w523, "Tree in"=w524) -> ("Tree Out"=w518:refnum<vi>)  [unwired: 5 in, 3 out]
            n401 = flat-sequence {
              tunnel: w518 -> [_]
              frame #0 {
                n402 = call "CRYUpdate Buttons.vi"() -> ()  [unwired: 12 in]
              }
            }
          }
        }
        n403 = case shown="True" w515 {
          tunnel: w514 -> [_ w528]
          tunnel: w511 -> [_ _]
          frame False {
          }
          frame True {
            n404 = property on="AxisChange" class="Bool (strict)"("Val(Sgnl)"=TRUE ("Value (Signaling)")) -> ()  [unwired: 2 in, 2 out]
            n405 = disable-structure shown="Disabled" {
              disable-tunnel: w528 -> [w530 _]
              frame Disabled {
                n406 = case shown="False" w530 {
                  frame False {
                    w531 = u32 0
                    n407 = property on="IntensityGraph" class="IntGraph (strict)"("BG Color"=w531, "FG Color"=w531) -> ()  [unwired: 2 in, 2 out]
                  }
                  frame True {
                  }
                }
              }
              frame Enabled {
              }
            }
          }
        }
      }
      event "Legend": Double Click {
        n408 = event-data() -> ("CtlRef"=w533:refnum<vi>, "Coords"=w532:T2)  [unwired: 8 out]
        n409 = disable-structure shown="Disabled" {
          disable-tunnel: w533 -> [w539 _]
          disable-tunnel: w532 -> [w538 _]
          frame Disabled {
            n410 = call "CRYGet MultiListBox Click State.vi"("Coords"=w538, "MultiList Box Ref In"=w539) -> ("State"=w537:bool)  [unwired: 6 in, 3 out]
            n411 = call "CRYClick Name in Legend.vi"("Mouse Point"=w538, "MCListbox Ref In"=w539) -> ("Active Row"=w535:i32, "Click State?"=w536:bool)  [unwired: 8 in]
            n412 = And(x=w537, y=w536) -> (x .and. y?=w534:bool)
            n413 = case shown="True" w534 {
              tunnel: w539 -> [_ w540]
              tunnel: w535 -> [_ w541]
              frame False {
              }
              frame True {
                n414 = call "CRYOpen Step by Legend.vi"("Active Row"=w541, "MCListbox Ref In"=w540, "Type"=enum16{"Curves", "Values", "Results", "WFM"}."WFM" ("Type In")) -> ()  [unwired: 9 in]
              }
            }
          }
          frame Enabled {
          }
        }
      }
      event "Legend": Mouse Move {
        n415 = event-data() -> ("Coords"=w550:T2)  [unwired: 5 out]
        n416 = control-ref of="Legend"() -> (w543:refnum<vi>)
        n417 = local read "TotalPlot"() -> (w549:u32)
        n418 = call "CRYData View Legend Mouse Move.vi"("TotalPlot"=w549, "Mouse Point"=w550, "MCListbox Ref In"=w543) -> ("CellSize"=w547:T10, "Position"=w546:T4, "Selected Row"=w545:i32, "Move State"=w544:bool, "CellBG"=w548:u32)  [unwired: 1 in, 3 out]
        n419 = case shown="True" w544 {
          tunnel: w548 -> [_ _]
          tunnel: w547 -> [_ _]
          tunnel: w546 -> [_ w553]
          tunnel: w545 -> [_ w555]
          frame False {
          }
          frame True {
            n420 = local write "OldRow"(w555) -> ()
            n421 = Subtract(x=w553, y=T4 {"Left"=8, "Top"=6}) -> (x-y=w551:T4)
            n422 = property on="Ramp" class="Ring (strict)"("Position"=w551, "Visible"=TRUE) -> ()  [unwired: 2 in, 2 out]
          }
        }
      }
      event "RemoveOne": Value Change {
        w563 = 0 ("Active X Scale")
        w562 = "" ("X Scale.Name Label.Text")
        n423 = event-data() -> ()  [unwired: 7 out]
        n424 = flat-sequence {
          tunnel: w556 -> [w568]
          tunnel: [w568] -> w557
          tunnel: w557 -> [w576]
          frame #0 {
            n425 = local read "CursorShow"() -> (w567:bool)
            n426 = case shown="True" w567 {
              tunnel: w568 -> [_ w571]
              frame False {
              }
              frame True {
                n427 = local read "Graph Number"() -> (w569:i32)
                n428 = Format Into String("DA_CUR_HIDE" ("input 1"), "AAA" ("input 2"), w569, 0 ("input 3")) -> (resulting string=w573:string)  [unwired: 3 in, 1 out]
                n429 = Enqueue Element(queue=w571, element=w573) -> ()  [unwired: 1 in, 4 out]
              }
            }
          }
          frame #1 {
            n430 = local read "PreviewShow"() -> (w575:bool)
            n431 = case shown="True" w575 {
              tunnel: w576 -> [_ w579]
              frame False {
              }
              frame True {
                n432 = local read "Graph Number"() -> (w577:i32)
                n433 = Format Into String("DA_PRE_HIDE" ("input 1"), "AAA" ("input 2"), w577, 0 ("input 3")) -> (resulting string=w581:string)  [unwired: 3 in, 1 out]
                n434 = Enqueue Element(queue=w579, element=w581) -> ()  [unwired: 1 in, 4 out]
              }
            }
          }
        }
        n435 = local write "TotalPlot"(u32 0 ("TotalPlot")) -> ()
        n436 = local write "OldRow"(-1 ("OldRow 2")) -> ()
        n437 = flat-sequence {
          frame #0 {
            n438 = control-ref of="This VI"() -> (w584:refnum<vi>)
            n439 = Build Array(-1 ("nData")) -> (w585:i32[])
            n440 = call "CRYSymbol Conversion.vi"("pGraph VI"=w584, "nDatas"=w585, "sActin"="LEGEND_REMOVE") -> ()  [unwired: 9 in]
          }
          frame #1 {
            n441 = control-ref of="Legend"() -> (w588:refnum<vi>)
            n442 = call "CRYData View Legend Item Delete.vi"("RowNumber"=-1, "Legend MultiListbox In"=w588) -> ()  [unwired: 10 out]
          }
        }
        n443 = property on="Ramp" class="Ring (strict)"("Visible"=FALSE) -> ()  [unwired: 2 in, 2 out]
        n444 = local write "CursorEnabled"(FALSE ("CursorEnabled")) -> ()
        n445 = local write "IntensityGraph"(dbl[][] [] ("Graph")) -> ()
        n446 = property on="IntensityGraph" class="IntGraph (strict)"("ActXScl"=w563, "XScale.NameLbl.Text"=w562, "ActYScl"=w563, "YScale.NameLbl.Text"=w562) -> ()  [unwired: 2 in, 2 out]
        n447 = property on="PreviewGraph" class="WFGraph (strict)"("ActXScl"=0 ("Active X Scale"), "XScale.ScaleFit"=u8 2 ("X Scale.Scale Fit")) -> ()  [unwired: 2 in, 2 out]
      }
      event "AxisChange": Value Change {
        n448 = event-data() -> ()  [unwired: 7 out]
        n449 = control-ref of="Legend"() -> (w590:refnum<vi>)
        n450 = call "CRYGet Legend Name.vi"("MCListbox Refnum"=w590) -> ("Names Out"=w589:string[])  [unwired: 10 in]
        n451 = Index Array(array=w589) -> (element=w595:string)  [unwired: 1 in]
        n452 = call "CRYGet Curve Library Data.vi"("Type"=enum16{"Curves", "Values", "Results", "WFM"}."WFM", "Data Name"=w595) -> ("Wave"=w593:T11)  [unwired: 4 out]
        n453 = Array Size(array=w589) -> (size(s)=w592:i32)
        n454 = Unbundle By Name(w593) -> ("X unit"=w594:string, "Y unit"=w591:string)
        n455 = case shown="0" w592 {
          tunnel: w594 -> [_ w600]
          tunnel: w591 -> [_ w599]
          frame 0 {
            w598 = 0 ("Active X Scale")
            w597 = "" ("X Scale.Name Label.Text")
            n456 = property on="IntensityGraph" class="IntGraph (strict)"("ActXScl"=w598, "XScale.NameLbl.Text"=w597, "ActYScl"=w598, "YScale.NameLbl.Text"=w597) -> ()  [unwired: 2 in, 2 out]
          }
          frame Default {
            n457 = property on="IntensityGraph" class="IntGraph (strict)"("ActXScl"=0 ("Active X Scale"), "XScale.NameLbl.Text"=w600, "ActYScl"=0 ("Active Y Scale"), "YScale.NameLbl.Text"=w599) -> ()  [unwired: 2 in, 2 out]
          }
        }
      }
      event "Ramp": Mouse Down? {
        n458 = event-data() -> ()  [unwired: 9 out]
        n459 = event-data("Button"=u16 2) -> ()  [unwired: 1 in, 1 out]
      }
      event "Ramp": Shortcut Menu Activation? {
        n460 = event-data() -> ("MenuRef"=w610:refnum<k9>)  [unwired: 7 out]
        n461 = Delete Menu Items(9:w610) -> (3:w612:refnum<k9>)  [unwired: 3 in, 1 out]
        n462 = call "CRYGet Window Menu.vi"("Tags"=string[] ["DA_INS_FIRE", "DA_INS_RAINBOW", "DA_INS_LOGUP", "DA_INS_LOGDOWN", "DA_INS_COLOUR", "DA_INS_ICE"]) -> ("Tags_Out"=w604:string[], "Names_Out"=w607:string[])  [unwired: 8 in, 1 out]
        n463 = Insert Menu Items(7:w604, 8:w607, 9:w612) -> (3:w605:refnum<k9>)  [unwired: 3 in, 2 out]
        n464 = property on="Ramp" class="Ring (strict)"() -> ("Value"=w606:u16)  [unwired: 2 in, 2 out]
        n465 = Index Array(array=w604, index=w606) -> (element=w609:string)
        n466 = Set Menu Item Info(6:TRUE ("checked"), 7:w609, 11:w605) -> ()  [unwired: 2 in, 4 out]
        n467 = event-data() -> ()  [unwired: 2 in, 1 out]
      }
      event "Ramp": Shortcut Menu Selection (User) {
        n468 = event-data() -> ("ItemTag"=w613:string)  [unwired: 8 out]
        n469 = flat-sequence {
          tunnel: w613 -> [w617]
          frame #0 {
            n470 = case shown="\"DA_INS_FIRE\", Default" w617 {
              tunnel: [u16 0 ("Ramp") u16 1 ("Ramp") u16 2 ("Ramp") u16 3 ("Ramp") u16 4 ("Ramp") u16 5 ("Ramp")] -> w614
              frame "DA_INS_FIRE", Default {
              }
              frame "DA_INS_RAINBOW" {
              }
              frame "DA_INS_LOGUP" {
              }
              frame "DA_INS_LOGDOWN" {
              }
              frame "DA_INS_COLOUR" {
              }
              frame "DA_INS_ICE" {
              }
            }
            n471 = local read "Intensity Property"() -> (w616:T1)
            n472 = property on="Ramp" class="Ring (strict)"("Value"=w614) -> ()  [unwired: 2 in, 2 out]
            n473 = Bundle By Name(cluster=w616, "Map Type"=w614) -> (w615:T1)
            n474 = local write "Intensity Property"(w615) -> ()
          }
          frame #1 {
            n475 = control-ref of="This VI"() -> (w624:refnum<vi>)
            n476 = call "CRYGet Graph Data.vi"("pGraph VI"=w624) -> ("Rows"=w625:i32[])  [unwired: 2 in, 8 out]
            n477 = call "CRYPlot Intensity Graph.vi"("pGraph VI In"=w624, "Selected Rows In"=w625) -> ()  [unwired: 6 in, 4 out]
          }
        }
      }
      event "RampShow": Value Change {
        n478 = event-data() -> ()  [unwired: 7 out]
        n479 = local read "Intensity Property"() -> (w627:T1)
        n480 = property on="Legend" class="MCListbox (strict)"("ActiveCell"=T5 {"Row"=0, "Column"=1} ("Active Cell:Active Cell")) -> ("ActiveCellPos"=w632:T4)  [unwired: 2 in, 2 out]
        n481 = Unbundle By Name(w627) -> ("Map Type"=w626:T7)
        n482 = Subtract(x=w632, y=T4 {"Left"=8, "Top"=6}) -> (x-y=w630:T4)
        n483 = property on="Ramp" class="Ring (strict)"("Position"=w630, "Value"=w626, "Visible"=TRUE) -> ()  [unwired: 2 in, 2 out]
      }
      event "IntensityGraph": Drag Enter {
        n484 = event-data() -> ("Available Data Names"=w633:string[])  [unwired: 1 out]
        n485 = disable-structure shown="Disabled" {
          disable-tunnel: [w636 TRUE] -> w634
          disable-tunnel: w633 -> [w635 _]
          frame Disabled {
            n486 = Search 1D Array(1D array=w635, element="CRY_GRAPH_DATA") -> (index of element=w638:i32)  [unwired: 1 out]
            n487 = Not Equal?(x=w638, y=-1) -> (x != y?=w636:bool)
          }
          frame Enabled {
          }
        }
        n488 = event-data("Accepted?"=w634) -> ()  [unwired: 1 in, 1 out]
      }
      event "IntensityGraph": Drop {
        n489 = event-data() -> ()  [unwired: 2 out]
        n490 = local read "Event Name"() -> (w641:string)
        n491 = local read "TotalPlot"() -> (w646:u32)
        n492 = control-ref of="This VI"() -> (w642:refnum<vi>)
        n493 = call "CRYDrop Data in Same Graph.vi"("pGraph VI"=w642, "Queue"=w643, "Total Plot In"=w646, "sAction"=w641) -> ("Accepted?"=w644:bool, "Total Plot Out"=w645:u32)  [unwired: 3 in, 3 out]
        n494 = local write "TotalPlot"(w645) -> ()
        n495 = event-data("Accepted?"=w644) -> ()  [unwired: 1 in, 1 out]
      }
      event "IntensityGraph": Cursor Grab {
        n496 = event-data() -> ("CursIdx"=w647:i32)  [unwired: 1 out]
        n497 = flat-sequence {
          tunnel: w647 -> [w648]
          frame #0 {
            n498 = Equal To 0?(x=w648) -> (x = 0?=w649:bool)
            n499 = local write "NewCursIdx"(w648) -> ()
            n500 = Select(t=u32 1 ("OldCursIdx"), s=w649, f=u32 0 ("OldCursIdx")) -> (s? t:f=w652:u32)
            n501 = local write "OldCursIdx"(w652) -> ()
          }
          frame #1 {
            n502 = property on="CursorColor" class="Bool (strict)"("Val(Sgnl)"=TRUE ("Value (Signaling)")) -> ()  [unwired: 2 in, 2 out]
          }
        }
      }
      event "IntensityGraph": Cursor Move {
        n503 = event-data() -> ()  [unwired: 10 out]
        n504 = property on="CursorPlot" class="Bool (strict)"("Val(Sgnl)"=TRUE ("Value (Signaling)")) -> ()  [unwired: 2 in, 2 out]
      }
      event "ReportDrop": Value Change {
        n505 = event-data() -> ()  [unwired: 7 out]
        n506 = local read "Event Name"() -> (w655:string)
        n507 = local read "TotalPlot"() -> (w659:u32)
        n508 = control-ref of="This VI"() -> (w657:refnum<vi>)
        n509 = call "CRYDrop Data in Same Graph.vi"("pGraph VI"=w657, "Queue"=w656, "Total Plot In"=w659, "sAction"=w655) -> ("Total Plot Out"=w658:u32)  [unwired: 3 in, 4 out]
        n510 = local write "TotalPlot"(w658) -> ()
      }
      event "IntensityGraph": Scale Range Change {
        n511 = event-data() -> ("Kind"=w660:enum16{"X-Scale", "Y-Scale", "Z-Scale"})  [unwired: 8 out]
        n512 = case shown="\"X-Scale\", Default" w660 {
          frame "X-Scale", Default {
            w695 = u8 0 ("X Scale.Scale Fit")
            n513 = property on="IntensityGraph" class="IntGraph (strict)"("XScale.ScaleFit"=w695) -> ()  [unwired: 2 in, 2 out]
            n514 = property on="PreviewGraph" class="WFGraph (strict)"("XScale.ScaleFit"=w695) -> ()  [unwired: 2 in, 2 out]
          }
          frame "Y-Scale" {
            n515 = property on="IntensityGraph" class="IntGraph (strict)"("YScale.ScaleFit"=u8 0 ("Y Scale.Scale Fit")) -> ()  [unwired: 2 in, 2 out]
          }
        }
        n516 = disable-structure shown="Disabled" {
          frame Disabled {
            n517 = local read "PreviewShow"() -> (w661:bool)
            n518 = case shown="True" w661 {
              frame False {
              }
              frame True {
                n519 = property on="IntensityGraph" class="IntGraph (strict)"() -> ("XScale.Maximum"=w690:dbl, "XScale.Minimum"=w691:dbl)  [unwired: 2 in, 2 out]
                n520 = property on="PreviewGraph" class="WFGraph (strict)"() -> ("XScale.Maximum"=w671:dbl, "XScale.Minimum"=w665:dbl)  [unwired: 2 in, 2 out]
                n521 = Greater?(x=w665, y=w691) -> (0:w692:bool)
                n522 = Less?(x=w671, y=w690) -> (x < y?=w689:bool)
                n523 = Subtract(x=w671, y=w665) -> (x-y=w670:dbl)
                n524 = Select(t=w671, s=w689, f=w690) -> (s? t:f=w666:dbl)
                n525 = Select(t=w665, s=w692, f=w691) -> (s? t:f=w667:dbl)
                n526 = Subtract(x=w667, y=w665) -> (x-y=w664:dbl)
                n527 = Subtract(x=w666, y=w665) -> (x-y=w663:dbl)
                n528 = property on="PreviewGraph" class="WFGraph (strict)"("Active Cursor"=u32 0, "Cursor.Cursor X"=w667, "Active Cursor"=u32 1, "Cursor.Cursor X"=w666) -> (error out=w688:errorcluster)  [unwired: 2 in, 1 out]
                n529 = Divide(x=w664, y=w670) -> (x/y=w668:dbl)
                n530 = Divide(x=w663, y=w670) -> (x/y=w669:dbl)
                n531 = property on="Scrollbar" class="Scroll (strict)"() -> ("DocMax"=w677:dbl, "PageSize"=w683:dbl)  [unwired: 2 in, 2 out]
                n532 = Subtract(x=w668, y=w669) -> (x-y=w675:dbl)
                n533 = flat-sequence {
                  tunnel: w688 -> [_]
                  frame #0 {
                    n534 = control-ref of="This VI"() -> (w694:refnum<vi>)
                    n535 = call "CRYPlot Intensity Graph Preview.vi"("sOption"="Move", "IntensityGraph VI Ref"=w694) -> ()  [unwired: 10 in]
                  }
                }
                n536 = Divide(x=w683, y=w675) -> (x/y=w674:dbl)
                n537 = local read "ScaleMax"() -> (w673:dbl)
                n538 = local read "ScaleMin"() -> (w672:dbl)
                n539 = Add(x=w677, y=w674) -> (x+y=w676:dbl)
                n540 = property on="Scrollbar" class="Scroll (strict)"("DocMin"=w676) -> ("DocMax"=w685:dbl, "DocMin"=w684:dbl)  [unwired: 2 in, 2 out]
                n541 = Subtract(x=w673, y=w672) -> (x-y=w662:dbl)
                n542 = Subtract(x=w668, y=w672) -> (x-y=w678:dbl)
                n543 = Subtract(x=w685, y=w684) -> (x-y=w679:dbl)
                n544 = Multiply(x=w678, y=w679) -> (x*y=w680:dbl)
                n545 = Divide(x=w680, y=w662) -> (x/y=w681:dbl)
                n546 = Add(x=w681, y=w684) -> (x+y=w682:dbl)
                n547 = property on="Scrollbar" class="Scroll (strict)"("Value"=w682) -> ()  [unwired: 2 in, 2 out]
              }
            }
          }
          frame Enabled {
          }
        }
      }
      event "Repaint Watermark": Value Change {
        # "Repaint Watermark: 0-none, 1-Unit 1, 2-Unit 1 & 2"
        n548 = event-data() -> ("OldVal"=w698:i32, "NewVal"=w697:i32)  [unwired: 5 out]
        n549 = Not Equal?(x=w698, y=w697) -> (x != y?=w699:bool)
        n550 = local write "Repaint Watermark"(w697) -> ()
        n551 = case shown="True" w699 {
          tunnel: w698 -> [_ w705]
          tunnel: w697 -> [_ w704]
          frame False {
          }
          frame True {
            n552 = Equal To 0?(x=w705) -> (x = 0?=w709:bool)
            n553 = Equal?(x=w704, y=1) -> (x = y?=w710:bool)
            n554 = Equal?(x=w705, y=1) -> (x = y?=w703:bool)
            n555 = Equal To 0?(x=w704) -> (x = 0?=w702:bool)
            n556 = And(x=w703, y=w702) -> (x .and. y?=w701:bool)
            n557 = And(x=w709, y=w710) -> (x .and. y?=w707:bool)
            n558 = Or(x=w707, y=w701) -> (x .or. y?=w700:bool)
            n559 = case shown="False" w700 {
              frame False {
                n560 = property on="IntensityGraph" class="IntGraph (strict)"("PlotImages.Front"=picture data[5B] ("Plot Images:Front")) -> (error out=w712:errorcluster)  [unwired: 2 in, 1 out]
                n561 = local read "Event Name"() -> (w711:string)
                n562 = property on="IntensityGraph" class="IntGraph (strict)"(error in=w712) -> ("Plot Bounds"=w714:T9)  [unwired: 1 in, 2 out]
                n563 = call "CRYGetWaterMark.vi"("Type"=w711, "Plot Area Bounds"=w714) -> ("WaterMark Image"=w713:picture)  [unwired: 2 in, 7 out]
                n564 = property on="IntensityGraph" class="IntGraph (strict)"("PlotImages.Front"=w713) -> ()  [unwired: 2 in, 2 out]
              }
              frame True {
              }
            }
          }
        }
      }
      event "PreviewGraph": Cursor Move {
        n565 = event-data() -> ()  [unwired: 10 out]
        n566 = disable-structure shown="Disabled" {
          frame Disabled {
            n567 = property on="PreviewGraph" class="WFGraph (strict)"("Active Cursor"=u32 0, "Active Cursor"=u32 1) -> ("Cursor.Cursor X"=w747:dbl, "Cursor.Cursor X"=w748:dbl)  [unwired: 2 in, 2 out]
            n568 = property on="PreviewGraph" class="WFGraph (strict)"("XScale.ScaleFit"=u8 0 ("X Scale.Scale Fit")) -> ()  [unwired: 2 in, 2 out]
            n569 = property on="PreviewGraph" class="WFGraph (strict)"("ActXScl"=0 ("Active X Scale")) -> ("XScale.Maximum"=w726:dbl, "XScale.Minimum"=w725:dbl)  [unwired: 2 in, 2 out]
            n570 = control-ref of="This VI"() -> (w719:refnum<vi>)
            n571 = Greater?(x=w747, y=w748) -> (0:w731:bool)
            n572 = call "CRYPlot Intensity Graph Preview.vi"("sOption"="Move", "IntensityGraph VI Ref"=w719) -> ()  [unwired: 10 in]
            n573 = case shown="False" w731 {
              tunnel: w747 -> [w750 w752]
              tunnel: w748 -> [w749 w751]
              tunnel: [w750 w751] -> w718
              tunnel: [w749 w752] -> w727
              frame False {
              }
              frame True {
              }
            }
            n574 = Subtract(x=w726, y=w725) -> (x-y=w721:dbl)
            n575 = property on="IntensityGraph" class="IntGraph (strict)"("XScale.Minimum"=w718, "XScale.Maximum"=w727) -> ()  [unwired: 2 in, 2 out]
            n576 = Subtract(x=w718, y=w725) -> (x-y=w724:dbl)
            n577 = Subtract(x=w727, y=w725) -> (x-y=w722:dbl)
            n578 = Divide(x=w724, y=w721) -> (x/y=w723:dbl)
            n579 = Divide(x=w722, y=w721) -> (x/y=w720:dbl)
            n580 = property on="Scrollbar" class="Scroll (strict)"() -> ("DocMax"=w737:dbl, "PageSize"=w744:dbl)  [unwired: 2 in, 2 out]
            n581 = Subtract(x=w723, y=w720) -> (x-y=w735:dbl)
            n582 = Divide(x=w744, y=w735) -> (x/y=w734:dbl)
            n583 = local read "ScaleMax"() -> (w733:dbl)
            n584 = local read "ScaleMin"() -> (w732:dbl)
            n585 = Add(x=w737, y=w734) -> (x+y=w736:dbl)
            n586 = property on="Scrollbar" class="Scroll (strict)"("DocMin"=w736) -> ("DocMax"=w746:dbl, "DocMin"=w745:dbl)  [unwired: 2 in, 2 out]
            n587 = Subtract(x=w733, y=w732) -> (x-y=w741:dbl)
            n588 = Subtract(x=w723, y=w732) -> (x-y=w738:dbl)
            n589 = Subtract(x=w746, y=w745) -> (x-y=w739:dbl)
            n590 = Multiply(x=w738, y=w739) -> (x*y=w740:dbl)
            n591 = Divide(x=w740, y=w741) -> (x/y=w742:dbl)
            n592 = Add(x=w742, y=w745) -> (x+y=w743:dbl)
            n593 = property on="Scrollbar" class="Scroll (strict)"("Value"=w743) -> ()  [unwired: 2 in, 2 out]
          }
          frame Enabled {
          }
        }
      }
      event "PreviewGraph": Mouse Down {
        n594 = event-data() -> ("Coords"=w754:T2)  [unwired: 1 out]
        n595 = property on="PreviewGraph" class="WFGraph (strict)"() -> ("Plot Bounds"=w755:T9, "Width"=w753:u32)  [unwired: 2 in, 2 out]
        n596 = disable-structure shown="Disabled" {
          disable-tunnel: w755 -> [w767 _]
          disable-tunnel: w754 -> [w766 _]
          disable-tunnel: w753 -> [w765 _]
          frame Disabled {
            n597 = Unbundle By Name(w766) -> ("Horizontal"=w760:i32)
            n598 = To Long Integer(number=w765) -> (32bit integer=w757:i32)
            n599 = Unbundle By Name(w767) -> ("Left"=w764:i16)
            n600 = property on="PreviewGraph" class="WFGraph (strict)"("XScale.ScaleFit"=u8 0 ("X Scale.Scale Fit")) -> ()  [unwired: 2 in, 2 out]
            n601 = To Long Integer(number=w764) -> (32bit integer=w758:i32)
            n602 = Add(x=w758, y=w757) -> (x+y=w759:i32)
            n603 = Less?(x=w760, y=w758) -> (x < y?=w762:bool)
            n604 = Greater?(x=w760, y=w759) -> (0:w761:bool)
            n605 = Or(x=w762, y=w761) -> (x .or. y?=w763:bool)
            n606 = case shown="False" w763 {
              tunnel: w758 -> [w772 _]
              tunnel: w757 -> [w771 _]
              tunnel: w760 -> [w770 _]
              frame False {
                n607 = property on="PreviewGraph" class="WFGraph (strict)"("ActXScl"=0 ("Active X Scale")) -> ("XScale.Maximum"=w783:dbl, "XScale.Minimum"=w779:dbl)  [unwired: 2 in, 2 out]
                n608 = property on="PreviewGraph" class="WFGraph (strict)"("Active Cursor"=u32 0, "Active Cursor"=u32 1) -> ("Cursor.Cursor X"=w769:dbl, "Cursor.Cursor X"=w768:dbl)  [unwired: 2 in, 2 out]
                n609 = Subtract(x=w770, y=w772) -> (x-y=w786:i32)
                n610 = Divide(x=w786, y=w771) -> (x/y=w782:dbl)
                n611 = Subtract(x=w783, y=w779) -> (x-y=w778:dbl)
                n612 = Less Or Equal?(x=w769, y=w768) -> (x <= y?=w790:bool)
                n613 = Multiply(x=w782, y=w778) -> (x*y=w781:dbl)
                n614 = Subtract(x=w769, y=w768) -> (x-y=w777:dbl)
                n615 = flat-sequence {
                  tunnel: w791 -> [_]
                  tunnel: w779 -> [w797]
                  tunnel: w778 -> [w794]
                  frame #0 {
                    n616 = property on="PreviewGraph" class="WFGraph (strict)"("Active Cursor"=u32 0, "Active Cursor"=u32 1) -> ("Cursor.Cursor X"=w801:dbl, "Cursor.Cursor X"=w800:dbl)  [unwired: 2 in, 2 out]
                    n617 = Greater?(x=w801, y=w800) -> (0:w817:bool)
                    n618 = case shown="True" w817 {
                      tunnel: w801 -> [w821 w823]
                      tunnel: w800 -> [w820 w822]
                      tunnel: [w821 w822] -> w799
                      tunnel: [w820 w823] -> w798
                      frame False {
                      }
                      frame True {
                      }
                    }
                    n619 = Subtract(x=w799, y=w797) -> (x-y=w796:dbl)
                    n620 = Subtract(x=w798, y=w797) -> (x-y=w793:dbl)
                    n621 = Divide(x=w796, y=w794) -> (x/y=w795:dbl)
                    n622 = Divide(x=w793, y=w794) -> (x/y=w792:dbl)
                    n623 = property on="IntensityGraph" class="IntGraph (strict)"("XScale.Minimum"=w799, "XScale.Maximum"=w798) -> ()  [unwired: 2 in, 2 out]
                    n624 = property on="Scrollbar" class="Scroll (strict)"() -> ("DocMax"=w811:dbl, "PageSize"=w804:dbl)  [unwired: 2 in, 2 out]
                    n625 = Subtract(x=w795, y=w792) -> (x-y=w813:dbl)
                    n626 = local read "ScaleMax"() -> (w815:dbl)
                    n627 = local read "ScaleMin"() -> (w816:dbl)
                    n628 = Divide(x=w804, y=w813) -> (x/y=w814:dbl)
                    n629 = Add(x=w811, y=w814) -> (x+y=w812:dbl)
                    n630 = property on="Scrollbar" class="Scroll (strict)"("DocMin"=w812) -> ("DocMax"=w802:dbl, "DocMin"=w803:dbl)  [unwired: 2 in, 2 out]
                    n631 = Subtract(x=w815, y=w816) -> (x-y=w807:dbl)
                    n632 = Subtract(x=w795, y=w816) -> (x-y=w810:dbl)
                    n633 = Subtract(x=w802, y=w803) -> (x-y=w809:dbl)
                    n634 = Multiply(x=w810, y=w809) -> (x*y=w808:dbl)
                    n635 = Divide(x=w808, y=w807) -> (x/y=w806:dbl)
                    n636 = Add(x=w806, y=w803) -> (x+y=w805:dbl)
                    n637 = property on="Scrollbar" class="Scroll (strict)"("Value"=w805) -> ()  [unwired: 2 in, 2 out]
                  }
                }
                n638 = Absolute Value(x=w777) -> (abs(x)=w776:dbl)
                n639 = Add(x=w781, y=w779) -> (x+y=w780:dbl)
                n640 = Divide(x=w776, y=2.0) -> (x/y=w774:dbl)
                n641 = case shown="True" w790 {
                  tunnel: [w828 w836] -> w788
                  tunnel: w780 -> [w824 w833]
                  tunnel: w769 -> [w827 _]
                  tunnel: w768 -> [_ w832]
                  tunnel: w774 -> [w826 w835]
                  frame True {
                    n642 = Add(x=w827, y=w826) -> (x+y=w825:dbl)
                    n643 = Greater?(x=w825, y=w824) -> (0:w831:bool)
                    n644 = Select(t=u32 0 ("Active Cursor"), s=w831, f=u32 1) -> (s? t:f=w828:u32)
                  }
                  frame False {
                    n645 = Add(x=w832, y=w835) -> (x+y=w834:dbl)
                    n646 = Greater?(x=w834, y=w833) -> (0:w839:bool)
                    n647 = Select(t=u32 1 ("Active Cursor"), s=w839, f=u32 0) -> (s? t:f=w836:u32)
                  }
                }
                n648 = property on="PreviewGraph" class="WFGraph (strict)"("Active Cursor"=w788, "Cursor.Cursor X"=w780) -> (error out=w787:errorcluster)  [unwired: 2 in, 1 out]
                n649 = flat-sequence {
                  tunnel: w787 -> [w842]
                  tunnel: [w842] -> w791
                  frame #0 {
                    n650 = control-ref of="This VI"() -> (w841:refnum<vi>)
                    n651 = call "CRYPlot Intensity Graph Preview.vi"("sOption"="Move", "IntensityGraph VI Ref"=w841) -> ()  [unwired: 10 in]
                  }
                }
                n652 = property on="IntensityGraph" class="IntGraph (strict)"("XScale.ScaleFit"=u8 0 ("X Scale.Scale Fit")) -> ()  [unwired: 2 in, 2 out]
              }
              frame True {
              }
            }
          }
          frame Enabled {
          }
        }
      }
      event "PreviewShow": Value Change {
        n653 = event-data() -> ("NewVal"=w843:bool)  [unwired: 6 out]
        n654 = disable-structure shown="Disabled" {
          disable-tunnel: w843 -> [w844 _]
          frame Disabled {
            n655 = flat-sequence {
              tunnel: w844 -> [w849]
              frame #0 {
                n656 = Select(t="DA_PRE_VIEW", s=w849, f="DA_PRE_HIDE") -> (s? t:f=w848:string)
                n657 = control-ref of="This VI"() -> (w845:refnum<vi>)
                n658 = call "CRYPreview InsDel.vi"("Graph VI Ref"=w845, "sAction"=w848) -> ()  [unwired: 10 in]
              }
              frame #1 {
                n659 = property on="ToolbarUpdate" class="Bool (strict)"("Val(Sgnl)"=TRUE ("Value (Signaling)")) -> ()  [unwired: 2 in, 2 out]
              }
            }
          }
          frame Enabled {
          }
        }
      }
      event "Scrollbar": Value Change {
        n660 = event-data() -> ("NewVal"=w851:dbl)  [unwired: 6 out]
        n661 = disable-structure shown="Disabled" {
          disable-tunnel: w851 -> [w865 _]
          frame Disabled {
            n662 = local read "ScaleMax"() -> (w875:dbl)
            n663 = local read "ScaleMin"() -> (w876:dbl)
            n664 = property on="Scrollbar" class="Scroll (strict)"() -> ("DocMin"=w874:dbl, "DocMax"=w873:dbl)  [unwired: 2 in, 2 out]
            n665 = property on="PreviewGraph" class="WFGraph (strict)"("ActXScl"=0 ("Active X Scale")) -> ("XScale.Maximum"=w861:dbl, "XScale.Minimum"=w856:dbl)  [unwired: 2 in, 2 out]
            n666 = property on="PreviewGraph" class="WFGraph (strict)"("Active Cursor"=u32 0, "Active Cursor"=u32 1) -> ("Cursor.Cursor X"=w868:dbl, "Cursor.Cursor X"=w869:dbl)  [unwired: 2 in, 2 out]
            n667 = property on="PreviewGraph" class="WFGraph (strict)"("XScale.ScaleFit"=u8 0 ("X Scale.Scale Fit")) -> ()  [unwired: 2 in, 2 out]
            n668 = Subtract(x=w873, y=w874) -> (x-y=w880:dbl)
            n669 = Subtract(x=w875, y=w876) -> (x-y=w878:dbl)
            n670 = Subtract(x=w865, y=w874) -> (x-y=w877:dbl)
            n671 = Subtract(x=w868, y=w869) -> (x-y=w870:dbl)
            n672 = Multiply(x=w877, y=w878) -> (x*y=w879:dbl)
            n673 = Subtract(x=w861, y=w856) -> (x-y=w854:dbl)
            n674 = Absolute Value(x=w870) -> (abs(x)=w855:dbl)
            n675 = Divide(x=w879, y=w880) -> (x/y=w860:dbl)
            n676 = Divide(x=w855, y=w854) -> (x/y=w853:dbl)
            n677 = Less Or Equal To 0?(x=w870) -> (x <= 0?=w871:bool)
            n678 = Add(x=w853, y=w860) -> (x+y=w859:dbl)
            n679 = Multiply(x=w854, y=w860) -> (x*y=w857:dbl)
            n680 = Multiply(x=w854, y=w859) -> (x*y=w858:dbl)
            n681 = Add(x=w856, y=w858) -> (x+y=w863:dbl)
            n682 = Add(x=w856, y=w857) -> (x+y=w862:dbl)
            n683 = case shown="True" w871 {
              tunnel: w862 -> [w884 w889]
              tunnel: w863 -> [w883 w888]
              tunnel: [w885 w890] -> w872
              tunnel: [w884 w889] -> w881
              tunnel: [w883 w888] -> w882
              frame True {
                n684 = property on="PreviewGraph" class="WFGraph (strict)"("Active Cursor"=u32 0, "Cursor.Cursor X"=w884, "Active Cursor"=u32 1, "Cursor.Cursor X"=w883) -> (error out=w885:errorcluster)  [unwired: 2 in, 1 out]
              }
              frame False {
                n685 = property on="PreviewGraph" class="WFGraph (strict)"("Active Cursor"=u32 1, "Cursor.Cursor X"=w889, "Active Cursor"=u32 0, "Cursor.Cursor X"=w888) -> (error out=w890:errorcluster)  [unwired: 2 in, 1 out]
              }
            }
            n686 = property on="IntensityGraph" class="IntGraph (strict)"("XScale.Minimum"=w881, "XScale.Maximum"=w882) -> ()  [unwired: 2 in, 2 out]
            n687 = flat-sequence {
              tunnel: w872 -> [_]
              frame #0 {
                n688 = control-ref of="This VI"() -> (w894:refnum<vi>)
                n689 = call "CRYPlot Intensity Graph Preview.vi"("sOption"="Move", "IntensityGraph VI Ref"=w894) -> ()  [unwired: 10 in]
              }
            }
          }
          frame Enabled {
          }
        }
      }
      event "OpenProperty": Value Change {
        n690 = event-data() -> ()  [unwired: 7 out]
        n691 = flat-sequence {
          frame #0 {
            n692 = local read "PropertyTab"() -> (w895:string)
            n693 = control-ref of="This VI"() -> (w896:refnum<vi>)
            n694 = call "CRYGraph Property Window Main.vi"("TabName"=w895, "pGraph VI In"=w896) -> ()  [unwired: 1 in, 9 out]
          }
          frame #1 {
            n695 = local write "PropertyTab"("" ("PropertyTab")) -> ()
          }
        }
      }
      event "ToolbarUpdate": Value Change {
        n696 = event-data() -> ()  [unwired: 7 out]
        n697 = local read "Event Name"() -> (w898:string)
        n698 = case shown="Default" w898 {
          frame "ViewReport" {
          }
          frame Default {
            n699 = control-ref of="This VI"() -> (w900:refnum<vi>)
            n700 = call "CRYUpdate DataView Toolbar.vi"("pVI"=w900) -> ()  [unwired: 11 in]
            n701 = call "CRYPreUpdate Sequence.vi"("EventName"="CurLibUpdate") -> ()  [unwired: 15 in]
          }
        }
      }
    }
    n702 = global read "CRYMain Sub Window Global.vi" "gStop"() -> (w115:bool)
    n703 = Or(x=w115, y="stop") -> (x .or. y?=w111:bool)
  }
  n704 = flat-sequence {
    tunnel: w1 -> [_]
    frame #0 {
      n705 = local write "StateOut"(TRUE ("StateOut")) -> ()
    }
  }
